vi "Graphical Test Runner - Main UI - .vi"() -> ()   [LabVIEW 2017]
doc: "Copyright © 2005 James Kring, Inc. - All Rights Reserved"
uses:
  Graphical Test Runner Support/Graphical TestRunner Throber List Static.ctl
  Graphical Test Runner Support/Graphical TestRunner Throber List Animated.ctl
  Classes/TestResult/resultStatusChanged--Cluster.ctl
  Classes/TestResult/resultStatus--enum.ctl
  Graphical Test Runner Support/FailbarStatus--Enum.ctl
  <userlib>/_OpenG.lib/comparison/comparison.llb/I32 Changed__ogtk.vi
  <userlib>/_OpenG.lib/file/file.llb/Valid Path - Traditional__ogtk.vi
  <userlib>/_OpenG.lib/array/array.llb/Filter 1D Array (Path)__ogtk.vi
  <userlib>/_OpenG.lib/file/file.llb/Strip Path - Arrays__ogtk.vi
  JKI Reuse/Filter Error Codes (Array)__jki_lib_error_handling -- VI Tester.vi
  <userlib>/_OpenG.lib/array/array.llb/Filter 1D Array (String)__ogtk.vi
  <userlib>/_OpenG.lib/array/array.llb/Delete Elements from 1D Array (Path)__ogtk.vi
  <userlib>/_OpenG.lib/array/array.llb/Conditional Auto-Indexing Tunnel (Path)__ogtk.vi
  <userlib>/_OpenG.lib/array/array.llb/Sort 1D Array (String)__ogtk.vi
  <userlib>/_OpenG.lib/array/array.llb/Index 1D Array Elements (Path)__ogtk.vi
  JKI Reuse/Filter Error Codes (Scalar)__jki_lib_error_handling -- VI Tester.vi
  Graphical Test Runner Support/GraphicalTestRunner.lvlib
  Libraries/VITesterUtilities.lvlib
  <vilib>/Utility/NIReport.llb/NI_report.lvclass
  Classes/TestResult/TestResult.lvclass
panel:
  in  "API_TesterStatus":refnum<user-event>
  in  "API_CompleteTestReport":refnum<user-event>
  in  "API_TextTestRunner":refnum<class>
  in  "Save Report":bool
  in  "API_TestObject":refnum<class>
  in  "Collapse Item":bool
  in  "Expand Item":bool
  in  "Collapse Tree":bool
  in  "Expand Tree":bool
  in  "Reload":bool
  in  "API_RunAll":bool
  in  "Abort":bool
  in  "Run Single Test":bool
  in  "Run All":bool
  out "Static Throber":T1=1
  out "Animated Throber":T2=1
  out "Slide":dbl(slide) min=0.0 max=100.0 scale=0.0..100.0
  out "txtRuns:":string caption="Last Run:"
  out "txtPassed:":string caption="Passed:"
  out "txtFailed:":string caption="Failed:"
  out "txtSkipped":string caption="Skipped:"
  in  "Test Hierarchy Tree":string(tree)
  out "Detailed Status":string
  out "Simple Status":string="Initializing ..."
  # "Copyright © 2007 James Kring, Inc. All rights reserved.\n\nAuthor: Omar Mussa [omar.mussa@jameskring.com]\n\nThis library is provided \"AS IS\" ,WITHOUT WARRANTIES OR \nCONDITIONS OF ANY KIND, either express or implied.\n\nJames Kring, Inc. -- http://www.jameskring.com"
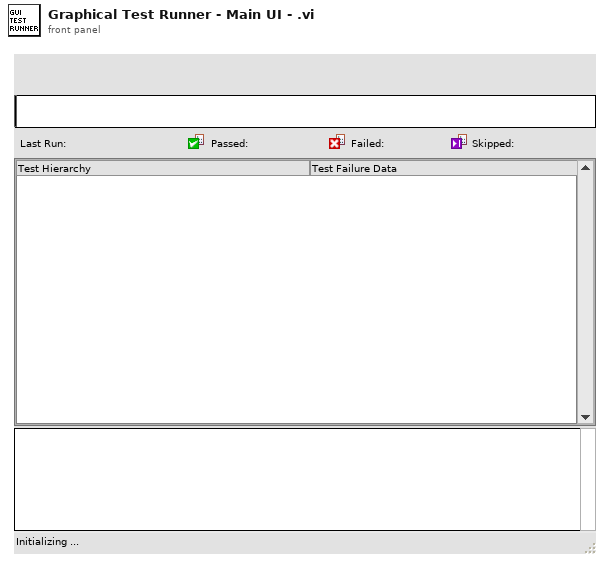
[diagram p1: front panel]
types:
  T1 = typedef "GraphicalTestRunner.lvlib/Graphical TestRunner Throber List Static.ctl" = u16
  T2 = typedef "GraphicalTestRunner.lvlib/Graphical TestRunner Throber List Animated.ctl" = u16
  T3 = typedef "TestResult.lvclass/resultStatusChanged--Cluster.ctl" = cluster{"test":refnum<class>, "resultStatus":T4, "TestResult":refnum<class>, "test error":errorcluster, "execution time (sec)":dbl}
  T4 = typedef "TestResult.lvclass/resultStatus--enum.ctl" = enum16{"testPass", "testFailure", "testError", "testSkipped"}
  T5 = cluster{"test":refnum<class>, "startTimestamp":timestamp}
  T6 = cluster{"Current VI's Refnum":refnum<vi>, "menubar":refnum<k9>, "TextStream":refnum<queue>, "StartTestTime":timestamp, "TestRunning":bool, "TestMethod":string, "Open Path":path, "Test Project":path, "TestProjectClasses":path[], "TestApplicationContext":refnum<vi>, "Test Class":path, "ResultChangedRef":refnum<user-event>, "SuiteChangedRef":refnum<user-event>, "TotalTests":i32, "TestTag":string, "Last Failure":string, "Last Tree Value":string, "AbortEventRef":refnum<user-event>, "TestMethods":path[], "ExitEventReference":refnum<user-event>, "InitializingTree":bool, "TestStartedEventRef":refnum<user-event>, "ProductName":string}
  T7 = cluster{"TestSuite":refnum<class>, "suiteStatus":enum16{"suiteStart", "suiteStop", "suiteSkip"}}
  T8 = enum8{"Enabled", "Disabled", "Disabled and Grayed Out"}
  T9 = enum32{"Invalid", "Standard", "Closed", "Hidden", "Minimized", "Maximized"}
  T10 = typedef "GraphicalTestRunner.lvlib/FailbarStatus--Enum.ctl" = enum16{"Initialize", "Start", "Update Progress", "Fail", "Pass"}
  T11 = cluster{"ResultStatusChanged":refnum<user-event>, "SuiteStatusChanged":refnum<user-event>, "Exit":refnum<user-event>, "Abort":refnum<user-event>, "TestStartedEventRef":refnum<user-event>}
  T12 = enum32{"existing file", "new file", "new or existing file", "existing dir", "new dir", "new or existing dir", "existing file (use LLBs)", "new file (use LLBs)", "new or existing file (use LLBs)", "new or existing file or directory (use LLBs)", "existing dir (use LLBs)", "new dir (use LLBs)", "new or existing dir (use LLBs)", "existing file or dir", "new file or dir", "new or existing file or dir", "existing file or dir (use LLBs)", "new file or dir (use LLBs)", "multi-select", "multi-select (use LLBs)"}
  T13 = typedef "LVPoint32TypeDef.ctl" = cluster{"Horizontal":i32, "Vertical":i32}
  T14 = cluster{"Recent Paths":path[], "SkipMassCompileCheck":bool}
  T15 = typedef "Filtered Error Details - Cluster__jki_lib_error_handling -- VI Tester.ctl" = cluster{"code":i32, "source":string}
  T16 = typedef "imagedata.ctl" = cluster{"image type":i32, "image depth":i32, "image":u8[], "mask":u8[], "colors":u32[], "Rectangle":cluster{"left":i16, "top":i16, "right":i16, "bottom":i16}}
  T17 = cluster{"txtRuns":refnum<vi>, "txtSkipped":refnum<vi>, "txtFailures":refnum<vi>, "txtPassed":refnum<vi>, "txtSimple Status":refnum<vi>, "Test Hierarchy Tree":refnum<vi>}
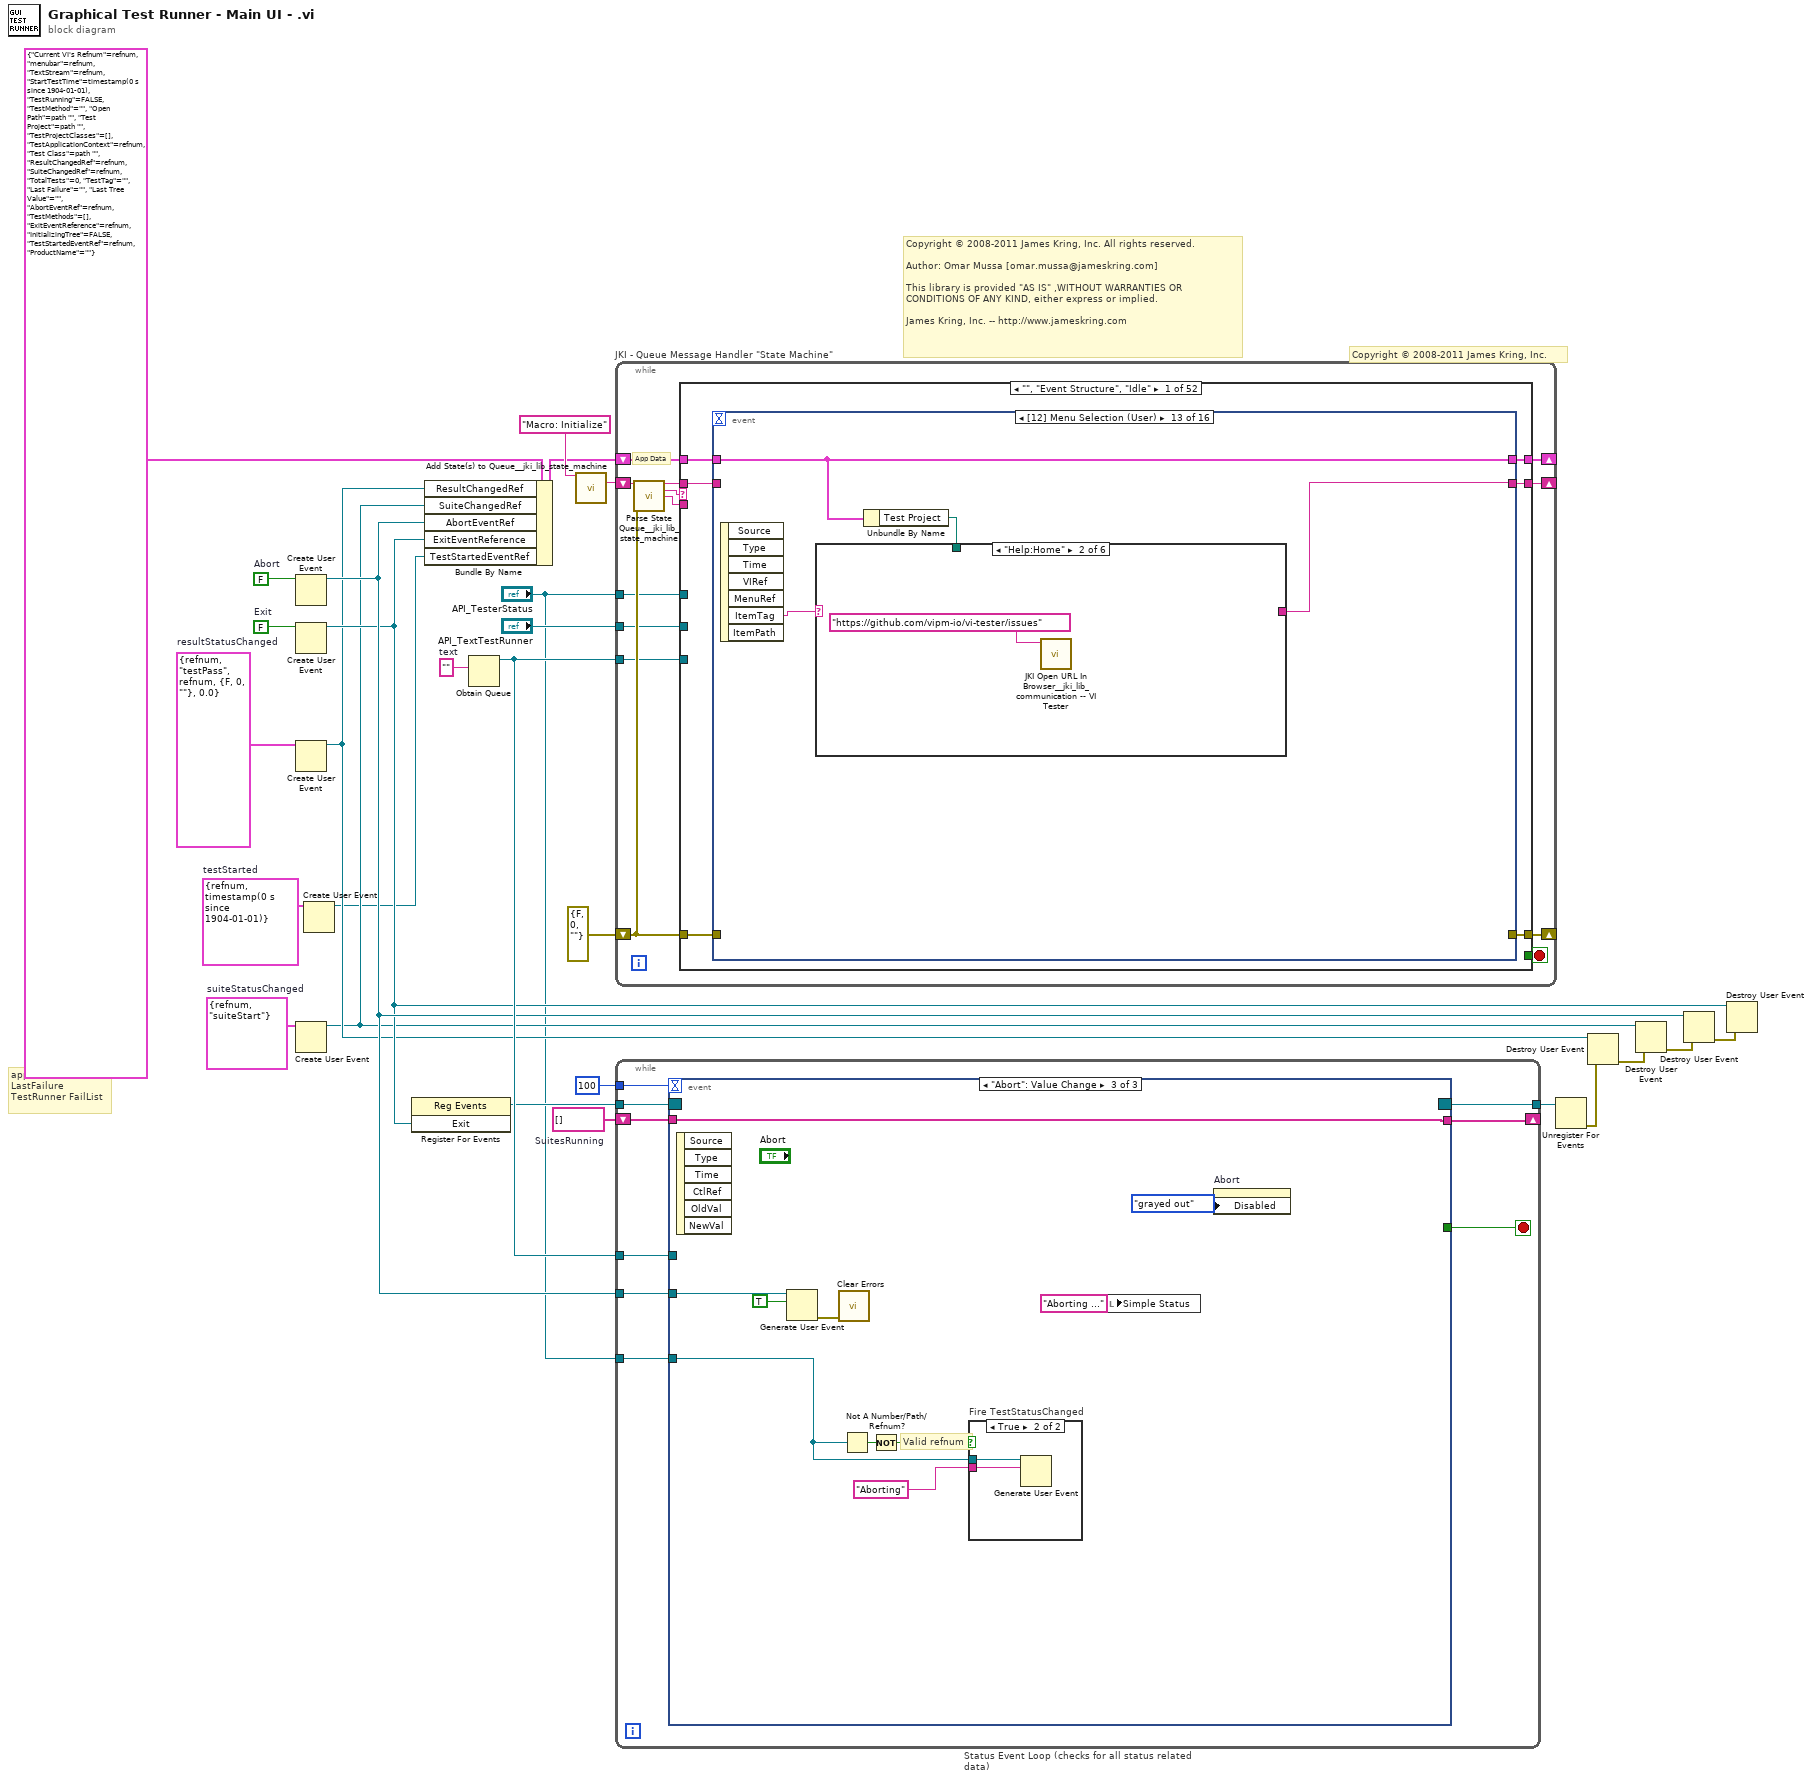
[diagram p0: block diagram]
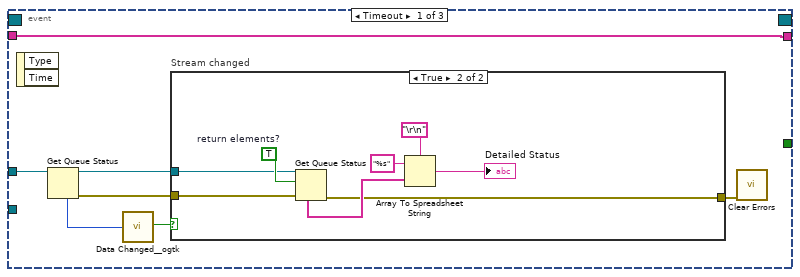
[diagram p2: hidden frame]
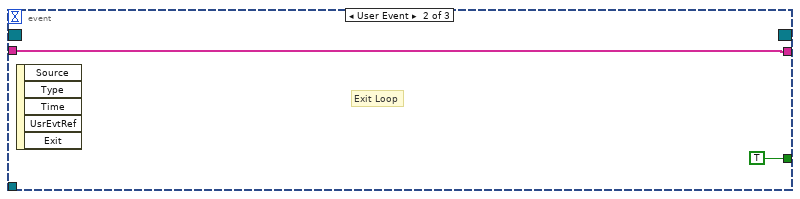
[diagram p4: hidden frame]
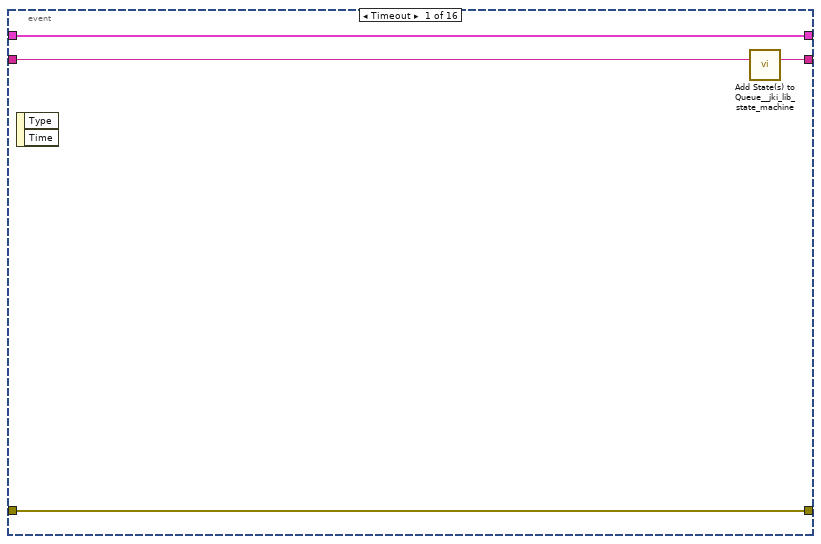
[diagram p6: hidden frame]
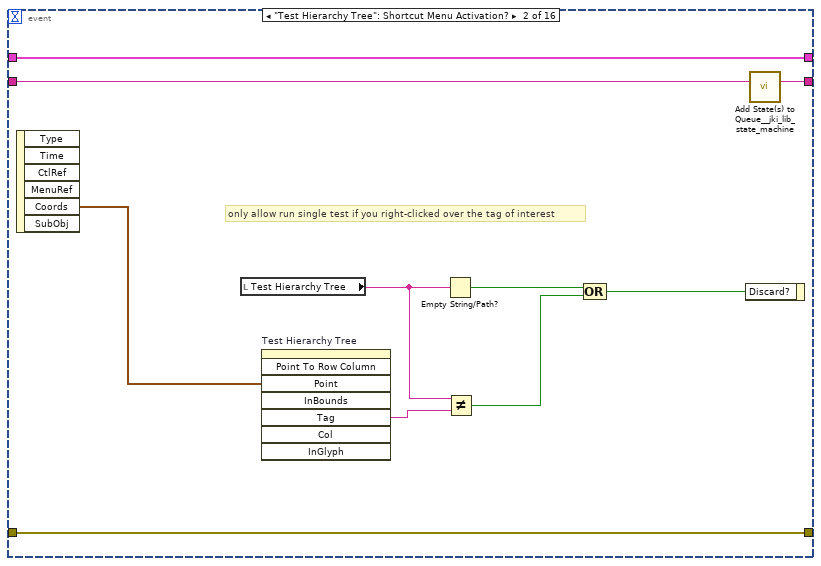
[diagram p7: hidden frame]
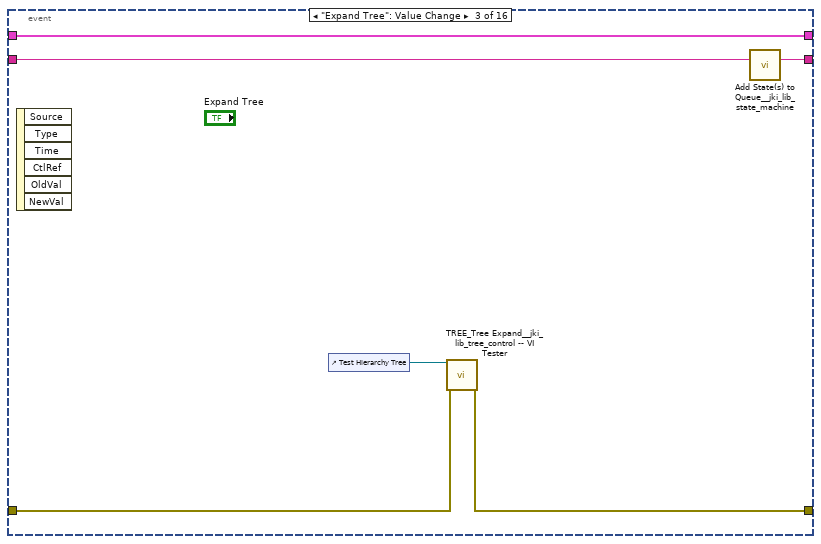
[diagram p8: hidden frame]
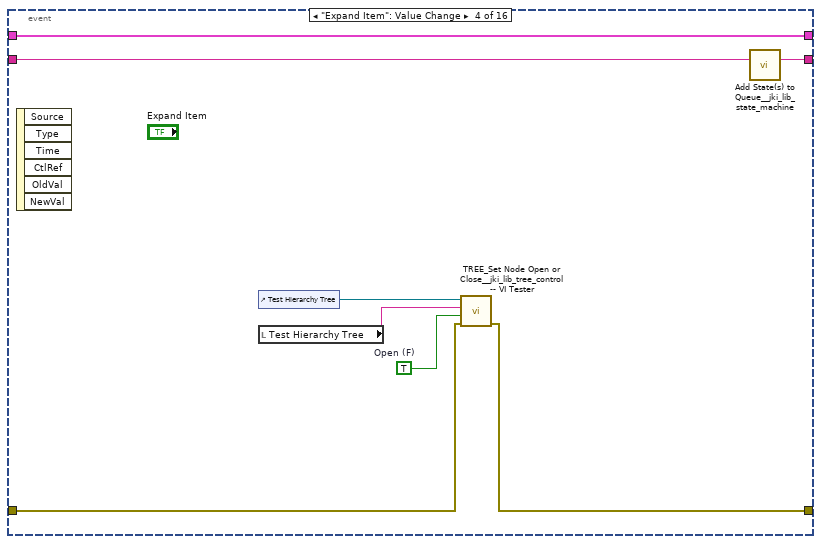
[diagram p9: hidden frame]
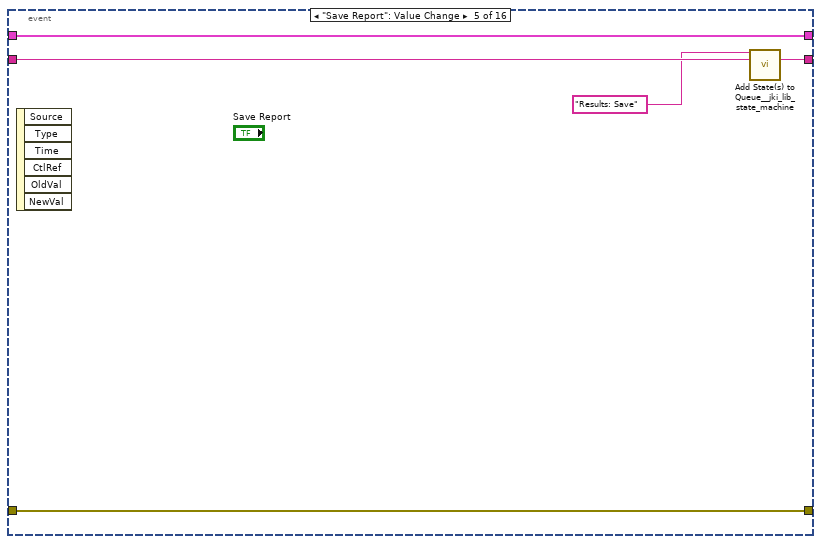
[diagram p10: hidden frame]
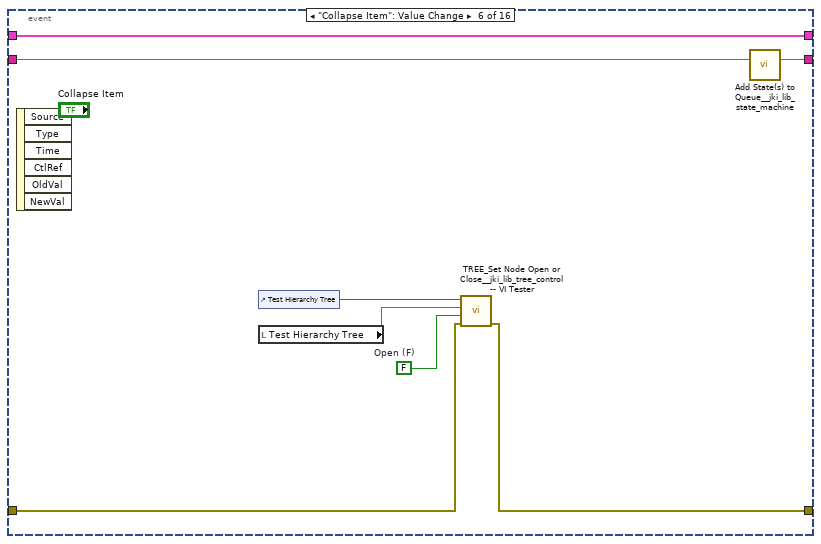
[diagram p11: hidden frame]
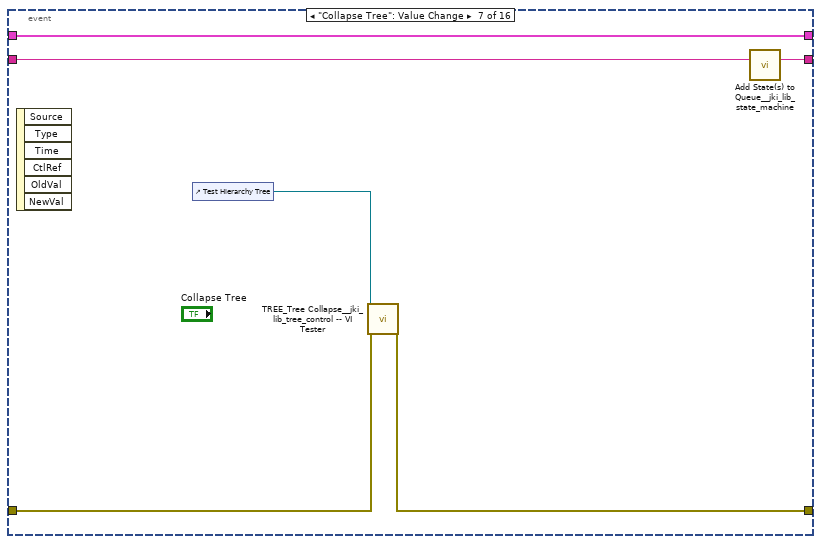
[diagram p12: hidden frame]
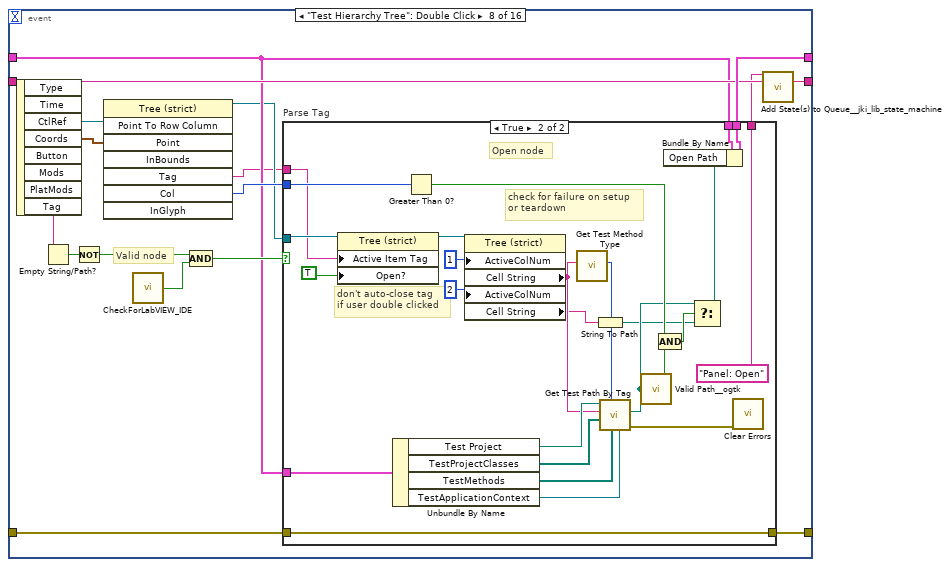
[diagram p13: hidden frame]
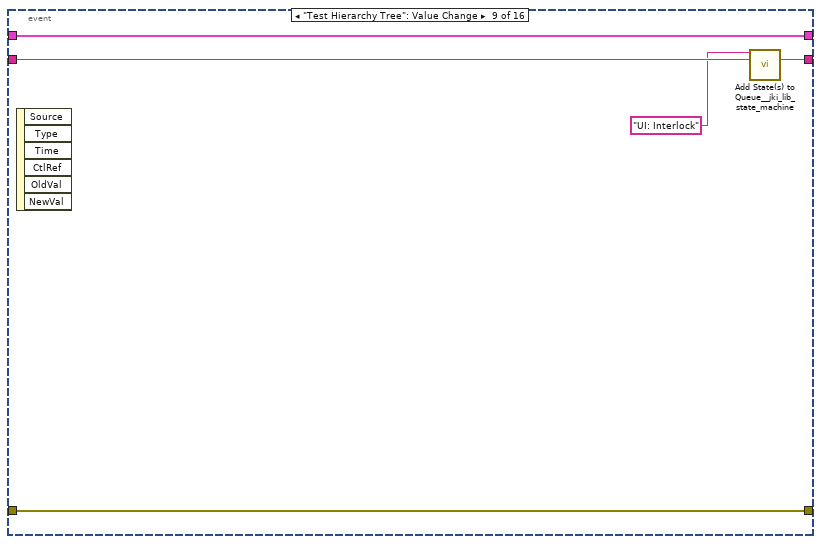
[diagram p15: hidden frame]
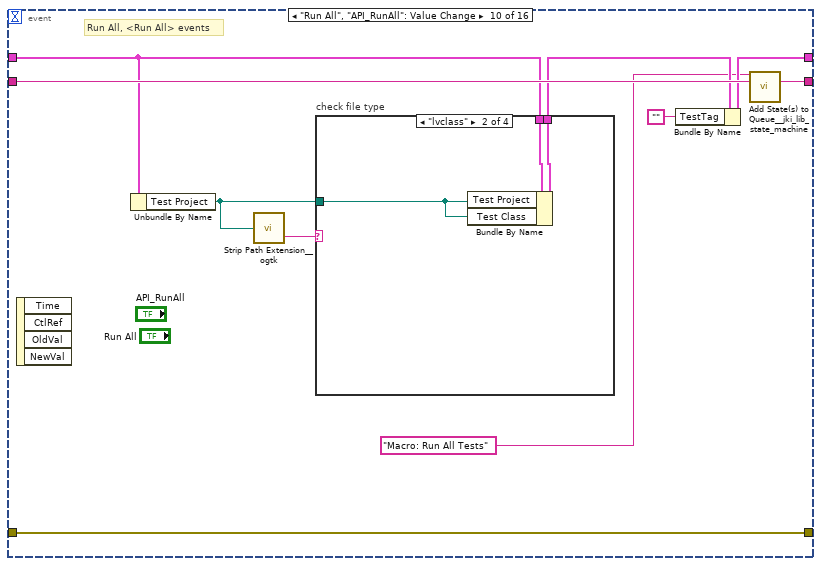
[diagram p16: hidden frame]
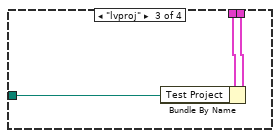
[diagram p18: hidden frame]
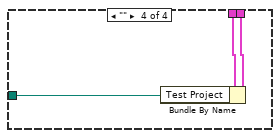
[diagram p19: hidden frame]
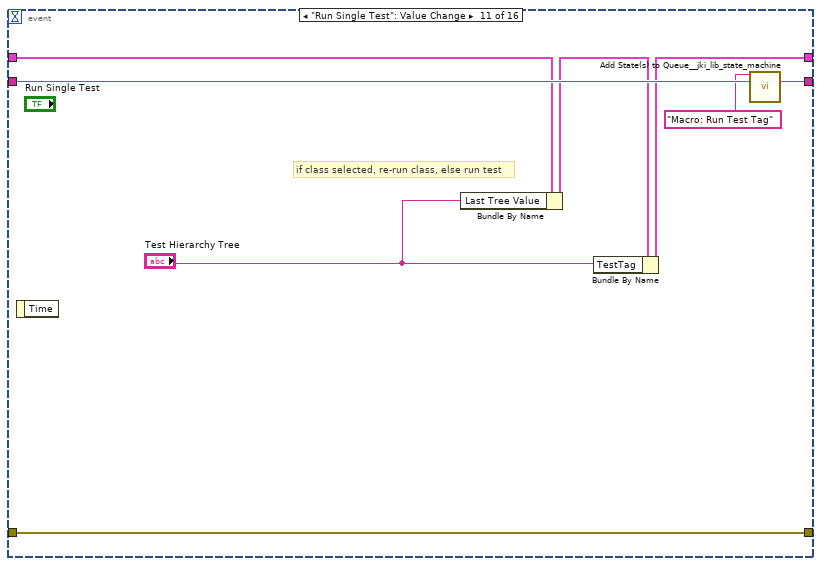
[diagram p20: hidden frame]
diagram:
  w2 = T3 {"test"=refnum, "resultStatus"=enum."testPass", "TestResult"=refnum, "test error"={"status"=FALSE, "code"=0, "source"=""}, "execution time (sec)"=0.0}  # resultStatusChanged
  w7 = T5 {"test"=refnum, "startTimestamp"=timestamp(0 s since 1904-01-01)}  # testStarted
  w8 = ""  # text
  w12 = FALSE  # Exit
  w16 = FALSE  # Abort
  w18 = string[] []  # SuitesRunning
  w19 = T7 {"TestSuite"=refnum, "suiteStatus"=enum."suiteStart"}  # suiteStatusChanged
  # "app data to delete\nLastFailure\nTestRunner FailList"
  # "Copyright © 2008-2011 James Kring, Inc. All rights reserved.\n\nAuthor: Omar Mussa [omar.mussa@jameskring.com]\n\nThis library is provided \"AS IS\" ,WITHOUT WARRANTIES OR \nCONDITIONS OF ANY KIND, either express or implied.\n\nJames Kring, Inc. -- http://www.jameskring.com"
  # "Copyright © 2008-2011 James Kring, Inc."
  n1 = Create User Event(user event datatype=w16) -> (user event=w13:refnum<user-event>)  [unwired: 1 in, 1 out]
  n2 = Create User Event(user event datatype=w12) -> (user event=w10:refnum<user-event>)  [unwired: 1 in, 1 out]
  n3 = Create User Event(user event datatype=w2) -> (user event=w6:refnum<user-event>)  [unwired: 1 in, 1 out]
  n4 = Create User Event(user event datatype=w19) -> (user event=w5:refnum<user-event>)  [unwired: 1 in, 1 out]
  n5 = Create User Event(user event datatype=w7) -> (user event=w4:refnum<user-event>)  [unwired: 1 in, 1 out]
  n6 = register-events(w10) -> (reference out=w22:refnum<event-registration>)  [unwired: 2 in, 1 out]
  n7 = Bundle By Name(cluster=T6 {"Current VI's Refnum"=refnum, "menubar"=refnum, "TextStream"=refnum, "StartTestTime"=timestamp(0 s since 1904-01-01), "TestRunning"=FALSE, "TestMethod"="", "Open Path"=path "", "Test Project"=path "", "TestProjectClasses"=[], "TestApplicationContext"=refnum, "Test Class"=path "", "ResultChangedRef"=refnum, "SuiteChangedRef"=refnum, "TotalTests"=0, "TestTag"="", "Last Failure"="", "Last Tree Value"="", "AbortEventRef"=refnum, "TestMethods"=[], "ExitEventReference"=refnum, "InitializingTree"=FALSE, "TestStartedEventRef"=refnum, "ProductName"=""} ("SMUI Template App Data"), "ResultChangedRef"=w6, "SuiteChangedRef"=w5, "AbortEventRef"=w13, "ExitEventReference"=w10, "TestStartedEventRef"=w4) -> (w23:T6)
  n8 = Obtain Queue(element data type=w8) -> (queue out=w24:refnum<queue>)  [unwired: 4 in, 2 out]
  n9 = call <vilib>:"Add State(s) to Queue__jki_lib_state_machine.vi"("State(s) in Front (\"\")"="Macro: Initialize") -> ("States Out"=w26:string)  [unwired: 14 in]
  n10 = while "JKI - Queue Message Handler \"State Machine\"" {
    shift-right: [w40] -> _
    shift-left: errorcluster {"status"=FALSE, "code"=0, "source"=""} ("error out") -> [w34]
    shift-right: [w38] -> _
    shift-left: w26 -> [w35]
    shift-right: [w36] -> _
    shift-left: w23 -> [w37]
    tunnel: w24 -> [w30]
    tunnel: "API_TextTestRunner" -> [w29]
    tunnel: "API_TesterStatus" -> [w28]
    stop <- w39 stop-if-true
    # "App Data"
    n11 = call <vilib>:"Parse State Queue__jki_lib_state_machine.vi"("State Queue"=w35, "Error In (no error)"=w34) -> ("Remaining States"=w33:string, "Current State"=w31:string, "Arguments"=w32:string)  [unwired: 11 in]
    n12 = case shown="\"\", \"Event Structure\", \"Idle\"" w31 {
      selector: w31 -> [_ _ w261 _ _ _ _ _ _ _ _ _ _ _ _ _ _ _ _ _ _ _ _ _ _ _ _ _ _ _ _ _ _ _ _ _ _ _ _ _ _ _ _ _ _ _ _ _ _ _ _ _]
      tunnel: w33 -> [w45 w252 w259 w270 w291 w305 w325 w333 w354 w357 w367 w376 w387 w405 w441 w447 w465 w477 w492 w523 w526 w537 w587 w609 w613 w628 w644 w659 w670 w680 w704 w723 w726 w734 w745 w756 w771 w804 w811 w828 w837 w842 w847 w857 w861 w872 w876 w889 w901 w910 w929 w939]
      tunnel: [w42 w254 w255 errorcluster {"status"=FALSE, "code"=0, "source"=""} ("error out") w293 w300 w327 w328 w334 w359 w361 w369 w378 w402 w442 w448 w467 w479 w494 w514 w528 w530 w589 w598 w610 w621 w629 w660 w667 w678 w688 w724 w728 w729 w735 w758 w767 w792 w813 w814 w839 w844 w849 w858 w863 w874 w878 w890 w903 w905 w918 w941] -> w40
      tunnel: w34 -> [w41 w254 _ w268 w293 w297 w327 w329 w334 w359 w361 w369 w383 w402 w442 w448 w467 w479 w494 w515 w528 w531 w589 w599 w610 w616 w630 w660 w666 w675 w682 w724 w728 w730 w735 w758 w769 w793 w813 w814 w839 w844 w849 w858 w863 w874 w878 w890 w903 w907 w919 w941]
      tunnel: [_ _ _ _ TRUE _ _ _ _ _ _ _ _ _ _ _ _ _ _ _ _ _ _ _ _ _ _ _ _ _ _ _ _ _ _ _ _ _ _ _ _ _ _ _ _ _ _ _ _ _ _ _] -> w39
      tunnel: [w46 w251 w260 w269 w291 w305 w324 w332 w353 w356 w366 w375 w386 w404 w440 w446 w466 w478 w493 w524 w525 w536 w586 w608 w612 w627 w643 w658 w669 w679 w703 w722 w725 w733 w744 w756 w770 w803 w810 w827 w836 w841 w846 w856 w860 w871 w875 w888 w900 w909 w928 w938] -> w38
      tunnel: w37 -> [w44 w253 w258 w263 w290 w299 w326 w331 w343 w358 w368 w377 w385 w406 w438 w445 w464 w476 w482 w522 w527 w533 w588 w600 w611 w614 w645 w655 w668 w673 w702 w715 w727 w732 w740 w757 w766 w801 w812 w826 w838 w843 w848 w855 w862 w873 w877 w884 w902 w911 w915 w940]
      tunnel: [w43 w253 w258 w263 w290 w299 w326 w331 w355 w358 w368 w377 w385 w406 w438 w445 w464 w476 w481 w522 w527 w533 w588 w600 w611 w626 w642 w655 w668 w673 w702 w721 w727 w732 w737 w757 w768 w802 w812 w818 w838 w843 w848 w855 w862 w873 w877 w883 w902 w911 w915 w940] -> w36
      tunnel: w32 -> [_ _ _ _ _ _ _ _ _ _ _ _ _ _ _ w444 _ _ _ _ _ _ _ _ _ _ _ w657 _ _ _ _ _ _ w743 _ _ _ _ _ _ _ _ _ _ _ _ _ _ _ _ _]
      tunnel: w30 -> [_ _ _ _ _ _ _ _ w344 _ _ _ _ _ _ _ w453 _ _ _ _ _ _ _ _ _ w635 _ _ _ w692 _ _ _ _ _ _ _ _ _ _ _ _ _ _ _ _ _ _ _ _ _]
      tunnel: w29 -> [_ _ _ _ _ _ _ _ _ _ _ _ _ _ _ _ _ _ _ _ _ _ _ _ _ w615 _ _ w665 w672 _ _ _ _ _ _ _ _ _ _ _ _ _ _ _ _ _ _ _ _ _ _]
      tunnel: w28 -> [_ _ _ _ _ _ _ _ _ _ _ _ _ _ _ _ _ _ _ _ _ _ _ _ _ _ w631 _ _ _ w684 _ _ _ _ _ _ _ _ _ _ _ _ _ _ _ _ _ _ _ _ _]
      frame "", "Event Structure", "Idle" {
        n13 = event shown="[12] Menu Selection (User)" {
          selector: _ -> [_ _ _ _ _ _ _ _ _ _ _ _ _ _ _ _]
          dyn-events: _ -> [_ _ _ _ _ _ _ _ _ _ _ _ _ _ _ _]
          timeout: _ -> [_ _ _ _ _ _ _ _ _ _ _ _ _ _ _ _]
          tunnel: [w49 w59 w65 w73 w78 w86 w92 w106 w142 w152 w170 w177 w186 _ w235 "Macro: Exit"] -> w46
          tunnel: w45 -> [w50 w60 w66 w74 w79 w87 w93 w107 w143 w153 w171 w178 _ _ _ _]
          tunnel: w44 -> [w48 w58 w64 w72 w77 w85 w91 w97 w141 w147 w165 w175 w184 w224 w233 w249]
          tunnel: [w48 w58 w64 w72 w77 w85 w91 w110 w141 w149 w169 w173 w184 w224 w232 w249] -> w43
          tunnel: [w47 w57 w61 w69 w76 w82 w88 w109 w140 w144 w167 w176 _ w220 _ _] -> w42
          tunnel: w41 -> [w47 w57 w62 w70 w76 w83 w89 w96 w140 w144 w167 w176 _ w222 _ _]
          event Timeout {
            n14 = event-data() -> ()  [unwired: 1 in, 2 out]
            n15 = call <vilib>:"Add State(s) to Queue__jki_lib_state_machine.vi"("State(s) in (\"\")"=w50) -> ("States Out"=w49:string)  [unwired: 14 in]
          }
          event "Test Hierarchy Tree": Shortcut Menu Activation? {
            # "only allow run single test if you right-clicked over the tag of interest"
            n16 = event-data() -> ("Coords"=w53:T13)  [unwired: 1 in, 5 out]
            n17 = local read "Test Hierarchy Tree"() -> (w51:string)
            n18 = invoke on="Test Hierarchy Tree" class="Tree (strict)" method="Point To Row Column"("Point"=w53) -> ("Tag"=w52:string)  [unwired: 7 in, 7 out]
            n19 = Empty String/Path?(string/path=w51) -> (empty?=w55:bool)
            n20 = Not Equal?(x=w51, y=w52) -> (x != y?=w56:bool)
            n21 = Compound Arithmetic op=OR(w55, w56) -> (w54:bool)
            n22 = event-data("Discard?"=w54) -> ()  [unwired: 1 in, 1 out]
            n23 = call <vilib>:"Add State(s) to Queue__jki_lib_state_machine.vi"("State(s) in (\"\")"=w60) -> ("States Out"=w59:string)  [unwired: 14 in]
          }
          event "Expand Tree": Value Change {
            n24 = event-data() -> ()  [unwired: 1 in, 6 out]
            n25 = control-ref of="Test Hierarchy Tree"() -> (w63:refnum<vi>)
            n26 = call "TREE_Tree Expand__jki_lib_tree_control -- VI Tester.vi"("Tree Reference In"=w63, "error in (no error)"=w62) -> ("error out"=w61:errorcluster)  [unwired: 16 in, 1 out]
            n27 = call <vilib>:"Add State(s) to Queue__jki_lib_state_machine.vi"("State(s) in (\"\")"=w66) -> ("States Out"=w65:string)  [unwired: 14 in]
          }
          event "Expand Item": Value Change {
            w67 = TRUE  # Open (F)
            n28 = event-data() -> ()  [unwired: 1 in, 6 out]
            n29 = control-ref of="Test Hierarchy Tree"() -> (w71:refnum<vi>)
            n30 = local read "Test Hierarchy Tree"() -> (w68:string)
            n31 = call "TREE_Set Node Open or Close__jki_lib_tree_control -- VI Tester.vi"("error in (no error)"=w70, "Open (F)"=w67, "Tag"=w68, "Tree Reference In"=w71) -> ("error out"=w69:errorcluster)  [unwired: 5 in, 2 out]
            n32 = call <vilib>:"Add State(s) to Queue__jki_lib_state_machine.vi"("State(s) in (\"\")"=w74) -> ("States Out"=w73:string)  [unwired: 14 in]
          }
          event "Save Report": Value Change {
            n33 = event-data() -> ()  [unwired: 1 in, 6 out]
            n34 = call <vilib>:"Add State(s) to Queue__jki_lib_state_machine.vi"("State(s) in Front (\"\")"="Results: Save" ("State(s) in Front (\"\")"), "State(s) in (\"\")"=w79) -> ("States Out"=w78:string)  [unwired: 13 in]
          }
          event "Collapse Item": Value Change {
            w80 = FALSE  # Open (F)
            n35 = event-data() -> ()  [unwired: 1 in, 6 out]
            n36 = control-ref of="Test Hierarchy Tree"() -> (w84:refnum<vi>)
            n37 = local read "Test Hierarchy Tree"() -> (w81:string)
            n38 = call "TREE_Set Node Open or Close__jki_lib_tree_control -- VI Tester.vi"("error in (no error)"=w83, "Open (F)"=w80, "Tag"=w81, "Tree Reference In"=w84) -> ("error out"=w82:errorcluster)  [unwired: 5 in, 2 out]
            n39 = call <vilib>:"Add State(s) to Queue__jki_lib_state_machine.vi"("State(s) in (\"\")"=w87) -> ("States Out"=w86:string)  [unwired: 14 in]
          }
          event "Collapse Tree": Value Change {
            n40 = event-data() -> ()  [unwired: 1 in, 6 out]
            n41 = control-ref of="Test Hierarchy Tree"() -> (w90:refnum<vi>)
            n42 = call "TREE_Tree Collapse__jki_lib_tree_control -- VI Tester.vi"("Tree Reference In"=w90, "error in (no error)"=w89) -> ("error out"=w88:errorcluster)  [unwired: 16 in, 1 out]
            n43 = call <vilib>:"Add State(s) to Queue__jki_lib_state_machine.vi"("State(s) in (\"\")"=w93) -> ("States Out"=w92:string)  [unwired: 14 in]
          }
          event "Test Hierarchy Tree": Double Click {
            # "Valid node"
            n44 = event-data() -> ("CtlRef"=w100:refnum<vi>, "Coords"=w99:T13, "Tag"=w101:string)  [unwired: 1 in, 5 out]
            n45 = Empty String/Path?(string/path=w101) -> (empty?=w108:bool)
            n46 = Not(x=w108) -> (.not. x?=w104:bool)
            n47 = invoke class="Tree (strict)" method="Point To Row Column"(reference=w100, "Point"=w99) -> (reference out=w95:refnum<vi>, "Tag"=w94:string, "Col"=w98:i32)  [unwired: 6 in, 5 out]
            n48 = call "CheckForLabVIEW_IDE.vi"() -> ("LabVIEW IDE"=w102:bool)
            n49 = Compound Arithmetic op=AND(w104, w102) -> (w103:bool)
            n50 = case "Parse Tag" shown="True" w103 {
              tunnel: [w111 w138] -> w110
              tunnel: [w112 w113] -> w109
              tunnel: w97 -> [w111 w137]
              tunnel: w96 -> [w112 w113]
              tunnel: [_ "Panel: Open" ("State(s) in Front")] -> w105
              tunnel: w98 -> [_ w135]
              tunnel: w95 -> [_ w120]
              tunnel: w97 -> [_ w133]
              tunnel: w94 -> [_ w117]
              frame False {
                # "Ignore double click if:\n1) Invalid node selected\n2) Running from Built EXE"
              }
              frame True {
                # "don't auto-close tag\nif user double clicked"
                # "check for failure on setup\nor teardown"
                # "Open node"
                n51 = property class="Tree (strict)"(reference=w120, "Active Item Tag"=w117, "Open?"=TRUE ("Active Item:Open?")) -> (reference out=w119:refnum<vi>)  [unwired: 1 in, 1 out]
                n52 = Unbundle By Name(w133) -> ("Test Project"=w132:path, "TestProjectClasses"=w129:path[], "TestMethods"=w128:path[], "TestApplicationContext"=w127:refnum<vi>)
                n53 = Greater Than 0?(x=w135) -> (x > 0?=w126:bool)
                n54 = property class="Tree (strict)"(reference=w119, "ActiveColNum"=1 ("Active Cell:Active Column Number"), "ActiveColNum"=2 ("Active Cell:Active Column Number")) -> ("Cell String"=w131:string, "Cell String"=w115:string)  [unwired: 1 in, 2 out]
                n55 = call "Get Test Method Type.vi"("Failure String"=w131) -> ("method type"=w130:enum16{"setUp", "testMethod", "tearDown"})  [unwired: 10 in]
                n56 = String To Path(string=w115) -> (path=w114:path)
                n57 = call "Get Test Path By Tag.vi"("TestApplicationContext"=w127, "TestMethods"=w128, "Method (testMethod)"=w130, "TestProjectClasses"=w129, "TestMethod Tag"=w131, "Test Project"=w132) -> ("error out"=w121:errorcluster, "Path"=w123:path)  [unwired: 2 in, 2 out]
                n58 = call-poly <userlib>:"Valid Path__ogtk.vi"("path"=w123) -> ("valid"=w125:bool)
                n59 = Compound Arithmetic op=AND(w126, w125) -> (w124:bool)
                n60 = Select(t=w123, s=w124, f=w114) -> (s? t:f=w122:path)
                n61 = Bundle By Name(cluster=w137, "Open Path"=w122) -> (w138:T6)
                n62 = call <vilib>:"Clear Errors.vi"("error in (no error)"=w121) -> ()  [unwired: 5 in, 2 out]
              }
            }
            n63 = call <vilib>:"Add State(s) to Queue__jki_lib_state_machine.vi"("State(s) in Front (\"\")"=w105, "State(s) in (\"\")"=w107) -> ("States Out"=w106:string)  [unwired: 13 in]
          }
          event "Test Hierarchy Tree": Value Change {
            n64 = event-data() -> ()  [unwired: 1 in, 6 out]
            n65 = call <vilib>:"Add State(s) to Queue__jki_lib_state_machine.vi"("State(s) in Front (\"\")"="UI: Interlock" ("State(s) in Front"), "State(s) in (\"\")"=w143) -> ("States Out"=w142:string)  [unwired: 13 in]
          }
          event "Run All", "API_RunAll": Value Change {
            # "Run All, <Run All> events"
            n66 = event-data() -> ()  [unwired: 1 in, 4 out]
            n67 = Unbundle By Name(w147) -> ("Test Project"=w145:path)
            n68 = call-poly <userlib>:"Strip Path Extension__ogtk.vi"("path"=w145) -> ("extension"=w150:string)  [unwired: 1 out]
            n69 = case "check file type" shown="\"lvclass\"" w150 {
              tunnel: w147 -> [w154 w157 w160 w163]
              tunnel: [w154 w156 w159 w162] -> w151
              tunnel: w145 -> [_ w155 w158 w161]
              frame Default {
              }
              frame "lvclass" {
                n70 = Bundle By Name(cluster=w157, "Test Project"=w155, "Test Class"=w155) -> (w156:T6)
              }
              frame "lvproj" {
                n71 = Bundle By Name(cluster=w160, "Test Project"=w158) -> (w159:T6)
              }
              frame "" {
                n72 = Bundle By Name(cluster=w163, "Test Project"=w161) -> (w162:T6)
              }
            }
            n73 = Bundle By Name(cluster=w151, "TestTag"="") -> (w149:T6)
            n74 = call <vilib>:"Add State(s) to Queue__jki_lib_state_machine.vi"("State(s) in Front (\"\")"="Macro: Run All Tests", "State(s) in (\"\")"=w153) -> ("States Out"=w152:string)  [unwired: 13 in]
          }
          event "Run Single Test": Value Change {
            # "if class selected, re-run class, else run test"
            n75 = event-data() -> ()  [unwired: 1 in, 1 out]
            n76 = Bundle By Name(cluster=w165, "Last Tree Value"="Test Hierarchy Tree") -> (w164:T6)
            n77 = Bundle By Name(cluster=w164, "TestTag"="Test Hierarchy Tree") -> (w169:T6)
            n78 = call <vilib>:"Add State(s) to Queue__jki_lib_state_machine.vi"("State(s) in Front (\"\")"="Macro: Run Test Tag", "State(s) in (\"\")"=w171) -> ("States Out"=w170:string)  [unwired: 13 in]
          }
          event "Test Hierarchy Tree": Shortcut Menu Selection (User) {
            n79 = event-data() -> ("ItemTag"=w174:string)  [unwired: 1 in, 5 out]
            n80 = case "Get Selected Method" shown="\"RunSingleTest\"" w174 {
              tunnel: w175 -> [w182 w183]
              tunnel: [w181 w183] -> w173
              tunnel: ["Macro: Run Test Tag" _] -> w172
              frame "RunSingleTest" {
                # "if class selected, re-run class, else run test"
                n81 = local read "Test Hierarchy Tree"() -> (w179:string)
                n82 = Bundle By Name(cluster=w182, "Last Tree Value"=w179, "TestTag"=w179) -> (w181:T6)
              }
              frame Default {
              }
            }
            n83 = call <vilib>:"Add State(s) to Queue__jki_lib_state_machine.vi"("State(s) in Front (\"\")"=w172, "State(s) in (\"\")"=w178) -> ("States Out"=w177:string)  [unwired: 13 in]
          }
          event Menu Selection (User) {
            n84 = event-data() -> ("ItemTag"=w187:string)  [unwired: 1 in, 6 out]
            n85 = Unbundle By Name(w184) -> ("Test Project"=w185:path)
            n86 = case shown="\"Help:Home\"" w187 {
              selector: w187 -> [w189 _ _ _ _ _]
              tunnel: [w190 _ _ "Macro: Exit" _ "UI: Open File Dialog"] -> w186
              tunnel: w185 -> [_ _ _ _ w201 _]
              frame Default {
                n87 = call <userlib>:"Search or Split String__ogtk.vi"("search string/char (-)"="Recent_Files:", "string"=w189) -> ("offset after match"=w192:i32, "substring after match"=w188:string)  [unwired: 1 in, 1 out]
                n88 = Greater Or Equal To 0?(x=w192) -> (x >= 0?=w191:bool)
                n89 = case shown="True" w191 {
                  tunnel: [w194 w195] -> w190
                  tunnel: w189 -> [w194 _]
                  tunnel: w188 -> [_ w197]
                  frame False {
                  }
                  frame True {
                    n90 = Format Into String(format string="Project: Open >> %s", w197) -> (resulting string=w195:string)  [unwired: 2 in, 1 out]
                  }
                }
              }
              frame "Help:Home" {
                n91 = call "JKI Open URL In Browser__jki_lib_communication -- VI Tester.vi"("url"="https://github.com/vipm-io/vi-tester/issues") -> ()  [unwired: 5 in, 2 out]
              }
              frame "About VI Tester..." {
                n92 = call "VI Tester About.vi"() -> ()  [unwired: 1 in]
              }
              frame "Exit" {
              }
              frame "Estimate Coverage..." {
                # "Estimate Test Coverage - Main UI - .vi"
                n93 = Build Path(base path=w201, name or relative path="..\\Tests") -> ()  [unwired: 1 out]
              }
              frame "File:Open_Project" {
              }
            }
          }
          event Menu Activation? {
            w217 = "Recent_Files" ("menu tag")
            # "Keep only if exists on disk"
            # "rebuild menu"
            # "flush existing menu"
            n94 = event-data() -> ("MenuRef"=w215:refnum<k9>)  [unwired: 1 in, 5 out]
            n95 = call "Read General Settings.vi"("error in"=w222) -> ("error out"=w211:errorcluster, "General"=w221:T14)  [unwired: 9 in]
            n96 = Unbundle By Name(w221) -> ("Recent Paths"=w205:path[])
            n97 = Build Array(path "", path "") -> (w208:path[])
            n98 = call-poly <userlib>:"Filter 1D Array__ogtk.vi"("items to filter"=w208, "array"=w205) -> ("filtered array"=w204:path[])  [unwired: 4 in, 1 out]
            n99 = for {
              tunnel: w204 -> [w228] mode=indexing
              tunnel: [w227] -> w203 mode=indexing if=w225
              n100 = call <vilib>:"Librarian Get Info.vi"("path"=w228) -> ("error out"=w226:errorcluster, "dup path"=w227:path)  [unwired: 8 in, 1 out]
              n101 = Not(x=w226) -> (.not. x?=w225:bool)
            }
            n102 = call-poly <userlib>:"Strip Path__ogtk.vi"("path"=w203) -> ("name"=w219:string[])  [unwired: 1 out]
            n103 = for {
              tunnel: w203 -> [w231] mode=indexing
              tunnel: [w230] -> w209 mode=indexing
              tunnel: "Recent_Files:%s" ("menu tag") -> [w229]
              n104 = Format Into String(format string=w229, w231) -> (resulting string=w230:string)  [unwired: 2 in, 1 out]
            }
            n105 = Get Menu Item Info(7:w217, 8:w211, 11:w215) -> (0:w212:errorcluster, 3:w214:refnum<k9>, 5:w216:string[])  [unwired: 4 out]
            n106 = Delete Menu Items(6:w212, 7:w216, 8:w217, 9:w214) -> (0:w210:errorcluster, 3:w213:refnum<k9>)
            n107 = Insert Menu Items(5:w217, 6:w210, 7:w209, 8:w219, 9:w213) -> (0:w220:errorcluster)  [unwired: 1 in, 2 out]
            n108 = event-data("Discard?"=FALSE) -> ()  [unwired: 1 in, 1 out]
          }
          event "Reload": Value Change {
            # "Reload"
            n109 = event-data() -> ()  [unwired: 1 in, 6 out]
            n110 = Unbundle By Name(w233) -> ("StartTestTime"=w236:timestamp)
            n111 = Not Equal?(x=timestamp(0 s since 1904-01-01) ("y"), y=w236) -> (x != y?=w238:bool)
            n112 = case "Test results exist" shown="True" w238 {
              tunnel: [TRUE ("T button?") w246] -> w234
              frame False {
              }
              frame True {
                n113 = Two Button Dialog(message="Reloading will clear the current results.", 2:"Reload" ("T button name (\"OK\")")) -> (T button?=w246:bool)  [unwired: 1 in]
              }
            }
            n114 = case shown="True" w234 {
              tunnel: [_ "UI: Set Busy\nMacro: Load Tree\nUI: Set Free" ("message")] -> w235
              tunnel: w233 -> [w239 w242]
              tunnel: [w239 w241] -> w232
              frame False {
              }
              frame True {
                n115 = Bundle By Name(cluster=w242, "StartTestTime"=timestamp(0 s since 1904-01-01)) -> (w241:T6)
              }
            }
          }
          event Panel Close? {
            n116 = event-data() -> ()  [unwired: 1 in, 4 out]
            n117 = event-data("Discard?"=TRUE) -> ()  [unwired: 1 in, 1 out]
          }
        }
      }
      frame "---------- Core ----------" {
        n118 = call <vilib>:"Add State(s) to Queue__jki_lib_state_machine.vi"("State(s) in (\"\")"=w252) -> ("States Out"=w251:string)  [unwired: 14 in]
      }
      frame Default {
        w257 = 42 items=["No error", "Argument error", "Memory is full", "Out of zone", "End of file", "File already open", "Generic file I/O error", "File not found", "File permission error", "Disk is full", "Duplicate path", "Too many files open", "System feature not enabled", "Resource file not found", "Cannot add resource", "Resource not found", "Image not found", "Image memory error", "Pen does not exist", "Config type invalid", "Config token not found", "Config parse error", "Config memory error", "Bad external code format", "Bad external code offset", "External code not present", "Null window", "Destroy window error", "Null menu", "Print aborted", "Bad print record", "Print driver error", "Windows error during printing", "Memory error during printing", "Print dialog error", "Generic print error", "Invalid device refnum", "Device not found", "Device parameter error", "Device unit error", "Cannot open device", "Device call aborted", "Generic error", "Cancelled by user", "Object ID too low", "Object ID too high", "Object not in heap", "Unknown heap", "Unknown object (invalid DefProc)", "Unknown object (DefProc not in table)", "Message out of range", "Invalid (null) method", "Unknown message", "Manager call not supported", "Bad address", "Network operation in progress", "Network operation timed out", "Connection is busy", "Network attribute not supported", "Network error", "Address in use", "System out of memory", "Connection aborted", "Connection refused", "Not connected", "Already connected", "Connection closed", "Initialization error (interapplication manager)", "Bad occurrence", "Wait on unbound occurrence handler", "Occurrence queue overflow", "Datalog type conflict", "Unused", "Unrecognized type (interapplication manager)", "Memory corrupt", "Failed to make temporary DLL", "Old CIN version", "Drag socket not found", "Failed to load drop-object", "Failed to register OLE object", "Failed to release OLE object", "Format specifier type mismatch", "Unknown format specifier", "Too few format specifiers", "Too many format specifiers", "Scan failed", "Newer CIN version", "Error converting to variant", "Runtime menu error", "Password tampered", "Variant attribute not found", "Incompatible variant data type", "Event data is not available", "Event Store is not present", "Occurrence is not found", "Event Queue is not created", "Event info is not available", "Refnum passed is NULL", "Error retrieving Class GUID", "Error retrieving CoClass GUID", "Error retrieving TypeLib GUID.", "Bad built application magic bytes.", "Specific driver is different from the specific driver associated with the Logical Name.", "There is no session opened to the class driver.", "Max Error", "MAX - Error with config objects", "MAX - Error loading configuration", "MAX - Group not supported"]
        n119 = Format Into String(format string="Software Exception: Unhandled State \"%s\"." ("message"), w261) -> (resulting string=w256:string)  [unwired: 2 in, 1 out]
        n120 = call <userlib>:"Build Error Cluster__ogtk.vi"("String to Prepend to source (\"\")"=w256, "code"=w257) -> ("error out"=w255:errorcluster)
        n121 = call <vilib>:"Add State(s) to Queue__jki_lib_state_machine.vi"("State(s) in (\"\")"=w259) -> ("States Out"=w260:string)  [unwired: 14 in]
      }
      frame "Error Handler" {
        n122 = call-poly "Filter Error Codes__jki_lib_error_handling -- VI Tester.vi"("error in"=w268, "error codes to filter"=i32[] [1448, 74]) -> ("error out"=w267:errorcluster, "error filtered?"=w266:bool, "filtered error details"=w264:T15)  [unwired: 7 in]
        n123 = case shown="False" w266 {
          tunnel: w267 -> [w272 _]
          tunnel: w264 -> [_ w275]
          tunnel: w263 -> [_ w273]
          frame False {
            # "Very simple Error Handler"
            n124 = call <vilib>:"General Error Handler.vi"("error in (no error)"=w272) -> ()  [unwired: 10 in, 5 out]
          }
          frame True {
            n125 = Unbundle By Name(w275) -> ("code"=w274:i32)
            n126 = case shown="Default" w274 {
              selector: w274 -> [_ _ w284]
              tunnel: ["One or more tests or test harnesses has an invalid connector pane.  Missing Test reference." w278 w283] -> w276
              tunnel: w273 -> [_ w279 _]
              frame 74 {
              }
              frame 1448 {
                n127 = Unbundle By Name(w279) -> ("Test Project"=w280:path)
                n128 = Format Into String(format string="Error: Could not load classes from '%s'.\nMake sure 1+ classes inherit from testCase or testSuite." ("message"), w280) -> (resulting string=w278:string)  [unwired: 2 in, 1 out]
              }
              frame Default {
                n129 = Format Into String(format string="Filtered error '%d' has undefined message!", w284) -> (resulting string=w283:string)  [unwired: 2 in, 1 out]
              }
            }
            n130 = One Button Dialog(message=w276) -> ()  [unwired: 1 in, 1 out]
          }
        }
        n131 = call <vilib>:"Add State(s) to Queue__jki_lib_state_machine.vi"("State(s) in (\"\")"=w270) -> ("States Out"=w269:string)  [unwired: 14 in]
      }
      frame "Exit" {
        # "Generate Exit Event to stop bottom loop"
        n132 = Unbundle By Name(w290) -> ("Current VI's Refnum"=w289:refnum<vi>, "ExitEventReference"=w287:refnum<user-event>)
        n133 = Close Reference(reference=w289) -> (error out=w288:errorcluster)  [unwired: 1 in]
        n134 = Generate User Event(user event=w287, event data cluster=TRUE ("event data")) -> (error out=w286:errorcluster)  [unwired: 2 in, 1 out]
        n135 = call <vilib>:"Clear Errors.vi"("error in (no error)"=w288) -> ()  [unwired: 5 in, 2 out]
        n136 = call <vilib>:"Clear Errors.vi"("error in (no error)"=w286) -> ()  [unwired: 5 in, 2 out]
      }
      frame "Self Mass Compile" {
        # "LabVIEW IDE"
        # "packaged"
        n137 = call "Graphical Test Runner - Get Version.vi"() -> ("Dev. Environment?"=w304:bool)  [unwired: 4 in, 1 out]
        n138 = call "CheckForLabVIEW_IDE.vi"() -> ("LabVIEW IDE"=w301:bool)
        n139 = call "Read General Settings.vi"("error in"=w297) -> ("error out"=w296:errorcluster, "General"=w295:T14)  [unwired: 9 in]
        n140 = Not(x=w304) -> (.not. x?=w303:bool)
        n141 = Unbundle By Name(w295) -> ("SkipMassCompileCheck"=w294:bool)
        n142 = Compound Arithmetic op=AND(w303, w301, invert w294) -> (w302:bool)
        n143 = Unbundle By Name(w299) -> ("ProductName"=w298:string)
        n144 = case "Built?  Mass Compile" shown="True" w302 {
          tunnel: w296 -> [w306 w313]
          tunnel: [w306 w314] -> w300
          tunnel: w298 -> [_ w307]
          frame False {
          }
          frame True {
            # "Force the VI Tester project provider VI tree to load, so it gets\nnoticed by the Mass Compile Tool, then unload it afterwards."
            n145 = call <userlib>:"Application Directory__ogtk.vi"("Relative path (.)"=path "resource/JKI/VI Tester") -> ("Application Directory (+ Relative)"=w321:path)
            n146 = call <userlib>:"Application Directory__ogtk.vi"("Relative path (.)"=path "vi.lib/addons/_JKI Toolkits/VI Tester") -> ("Application Directory (+ Relative)"=w320:path)
            n147 = call <userlib>:"Application Directory__ogtk.vi"("Relative path (.)"=path "resource/Framework/Providers/vitester") -> ("Application Directory (+ Relative)"=w318:path)
            n148 = Build Path(base path=w318, name or relative path="VITester - VI Tree.vi") -> (appended path=w316:path)
            n149 = Build Array(w321, w320, w318) -> (w310:path[])
            n150 = Open VI Reference(vi path=w316, error in (no error)=w313) -> (vi reference=w315:refnum<vi>, error out=w309:errorcluster)  [unwired: 4 in]
            n151 = call "Mass Compile LabVIEW Tool__jki_lib_application_control -- VI Tester.vi"("error in (no error)"=w309, "Product Folders"=w310, "Product Name"=w307) -> ("error out"=w308:errorcluster)  [unwired: 8 in]
            n152 = call "Clear All Errors__jki_lib_error_handling -- VI Tester.vi"("error in"=w308) -> ("no error out"=w311:errorcluster)  [unwired: 4 in]
            n153 = Close Reference(reference=w315, error in (no error)=w311) -> (error out=w312:errorcluster)
            n154 = Merge Errors(w308, w312) -> (w314:errorcluster)
          }
        }
      }
      frame "---------- App Data ----------" {
        n155 = call <vilib>:"Add State(s) to Queue__jki_lib_state_machine.vi"("State(s) in (\"\")"=w325) -> ("States Out"=w324:string)  [unwired: 14 in]
      }
      frame "App Data: Cleanup" {
        n156 = Unbundle By Name(w331) -> ("TextStream"=w330:refnum<queue>)
        n157 = Release Queue(queue=w330, error in (no error)=w329) -> (error out=w328:errorcluster)  [unwired: 1 in, 2 out]
        n158 = call <vilib>:"Add State(s) to Queue__jki_lib_state_machine.vi"("State(s) in (\"\")"=w333) -> ("States Out"=w332:string)  [unwired: 14 in]
      }
      frame "App Data: Initialize" {
        # "if TestObject is wired, use it to load project"
        # "ignore error if project not used to launch UI"
        # "This should eventually use the same app context (reference) as the project (or app menu) that was used to launch the GUI Test Runner."
        n159 = property class="App"() -> (error out=w347:errorcluster, "Project.ActiveProject"=w349:refnum<vi>)  [unwired: 2 in, 1 out]
        n160 = Equal?(x="API_TestObject", y=refnum<class> refnum ("TestObject In")) -> (x = y?=w341:bool)
        n161 = call <vilib>:"Get LV Class Path.vi"("object"="API_TestObject") -> ("error out"=w340:errorcluster, "class path"=w339:path)  [unwired: 9 in]
        n162 = property class="Project"(reference=w349, error in=w347) -> (reference out=w348:refnum<vi>, error out=w346:errorcluster, "Path"=w338:path)
        n163 = call <vilib>:"Clear Errors.vi"("error in (no error)"=w340) -> ()  [unwired: 5 in, 2 out]
        n164 = control-ref of="This Application"() -> (w350:refnum<vi>)
        n165 = Close Reference(reference=w348, error in (no error)=w346) -> (error out=w345:errorcluster)
        n166 = Select(t=w338, s=w341, f=w339) -> (s? t:f=w336:path)
        n167 = call <vilib>:"Clear Errors.vi"("error in (no error)"=w345) -> ()  [unwired: 5 in, 2 out]
        n168 = control-ref of="This VI"() -> (w352:refnum<vi>)
        n169 = Current VI's Menubar() -> (w351:refnum<k9>)
        n170 = Bundle By Name(cluster=w343, "TestApplicationContext"=w350, "Current VI's Refnum"=w352, "menubar"=w351, "TextStream"=w344, "Test Project"=w336, "ProductName"="VI Tester") -> (w355:T6)
        n171 = call <vilib>:"Add State(s) to Queue__jki_lib_state_machine.vi"("State(s) in (\"\")"=w354) -> ("States Out"=w353:string)  [unwired: 14 in]
      }
      frame "---------- UI ----------" {
        n172 = call <vilib>:"Add State(s) to Queue__jki_lib_state_machine.vi"("State(s) in (\"\")"=w357) -> ("States Out"=w356:string)  [unwired: 14 in]
      }
      frame "UI: Set Busy" {
        w363 = TRUE  # animate?
        n173 = control-ref of="This VI"() -> (w362:refnum<vi>)
        n174 = control-ref of="Animated Throber"() -> (w365:refnum<vi>)
        n175 = control-ref of="Static Throber"() -> (w364:refnum<vi>)
        n176 = call <vilib>:"Set Busy.vi"("VI reference (current VI)"=w362) -> ("error out"=w360:errorcluster)  [unwired: 9 in, 1 out]
        n177 = call "Throber Control__jki_lib_user_interface -- VI Tester.vi"("animate?"=w363, "static throber reference"=w364, "animate throber reference"=w365) -> ()  [unwired: 9 in]
        n178 = call <vilib>:"Clear Errors.vi"("error in (no error)"=w360) -> ()  [unwired: 5 in, 2 out]
        n179 = call <vilib>:"Add State(s) to Queue__jki_lib_state_machine.vi"("State(s) in (\"\")"=w367) -> ("States Out"=w366:string)  [unwired: 14 in]
      }
      frame "UI: Set Free" {
        w372 = FALSE  # animate?
        n180 = control-ref of="Animated Throber"() -> (w374:refnum<vi>)
        n181 = control-ref of="Static Throber"() -> (w373:refnum<vi>)
        n182 = call "Throber Control__jki_lib_user_interface -- VI Tester.vi"("animate?"=w372, "static throber reference"=w373, "animate throber reference"=w374) -> ()  [unwired: 9 in]
        n183 = control-ref of="This VI"() -> (w371:refnum<vi>)
        n184 = call <vilib>:"Unset Busy.vi"("VI reference (current VI)"=w371) -> ("error out"=w370:errorcluster)  [unwired: 10 in]
        n185 = call <vilib>:"Clear Errors.vi"("error in (no error)"=w370) -> ()  [unwired: 5 in, 2 out]
        n186 = call <vilib>:"Add State(s) to Queue__jki_lib_state_machine.vi"("State(s) in (\"\")"=w376) -> ("States Out"=w375:string)  [unwired: 14 in]
      }
      frame "UI: Reset Tree Status" {
        n187 = Unbundle By Name(w385) -> ("TestTag"=w382:string)
        n188 = control-ref of="Test Hierarchy Tree"() -> (w384:refnum<vi>)
        n189 = call "Get All.vi"("Tree Reference In"=w384, "Starting Tag"=w382, "error in (no error)"=w383) -> ("Tree Reference Out"=w380:refnum<vi>, "Output Tree Items"=w381:string[], "error out"=w379:errorcluster)  [unwired: 13 in, 1 out]
        n190 = for {
          tunnel: w381 -> [w391] mode=indexing
          tunnel: w380 -> [w394]
          shift-right: [w392] -> w378
          shift-left: w379 -> [w393]
          n191 = Match Pattern(string=w391, regular expression=".lvclass") -> (offset past match=w389:i32)  [unwired: 1 in, 3 out]
          n192 = Less Or Equal To 0?(x=w389) -> (x <= 0?=w388:bool)
          n193 = case "Init Test Icon" shown="True" w388 {
            tunnel: w394 -> [_ w399]
            tunnel: w393 -> [w395 w398]
            tunnel: [w395 w397] -> w392
            tunnel: w391 -> [_ w396]
            frame False {
              # "leave class icon alone"
            }
            frame True {
              w400 = 39  # custom VI index
              n194 = property class="Tree"(reference=w399, error in=w398, "Active Item Tag"=w396, "Glyph"=w400) -> (error out=w397:errorcluster)  [unwired: 1 out]
            }
          }
        }
        n195 = call <vilib>:"Add State(s) to Queue__jki_lib_state_machine.vi"("State(s) in (\"\")"=w387) -> ("States Out"=w386:string)  [unwired: 14 in]
      }
      frame "UI: Init Tree Symbols" {
        n196 = invoke on="Test Hierarchy Tree" class="Tree (strict)" method="Custom Item Symbols.Revert Symbols"() -> (error out=w403:errorcluster)  [unwired: 3 in, 2 out]
        n197 = call "Get Tree Symbols.vi"() -> ("Tree Symbols"=w401:T16[])  [unwired: 11 in]
        n198 = invoke on="Test Hierarchy Tree" class="Tree (strict)" method="Custom Item Symbols.Set Symbol Array"(error in=w403, "glyphs"=w401) -> ()  [unwired: 2 in, 4 out]
        n199 = call <vilib>:"Add State(s) to Queue__jki_lib_state_machine.vi"("State(s) in (\"\")"=w405) -> ("States Out"=w404:string)  [unwired: 14 in]
      }
      frame "UI: Interlock" {
        # "abort is only enabled when testSuite.run invoked"
        n200 = Unbundle By Name(w438) -> ("TestRunning"=w412:bool, "InitializingTree"=w407:bool)
        n201 = property on="Test Hierarchy Tree" class="Tree (strict)"() -> ("DispItems"=w434:string[])  [unwired: 2 in, 2 out]
        n202 = local read "Detailed Status"() -> (w414:string)
        n203 = property on="Test Hierarchy Tree" class="Tree (strict)"() -> ("DispItems"=w418:string[], "Value"=w417:string)  [unwired: 2 in, 2 out]
        n204 = Not(x=w407) -> (.not. x?=w422:bool)
        n205 = Not(x=w412) -> (.not. x?=w424:bool)
        n206 = property on="Abort" class="Bool"("Disabled"=enum16{"enabled", "disabled", "grayed out"}."grayed out") -> ()  [unwired: 2 in, 2 out]
        n207 = Empty String/Path?(string/path=w414) -> (empty?=w413:bool)
        n208 = Array Size(array=w418) -> (size(s)=w419:i32)
        n209 = Empty String/Path?(string/path=w417) -> (empty?=w416:bool)
        n210 = Greater Than 0?(x=w419) -> (x > 0?=w415:bool)
        n211 = Array Size(array=w434) -> (size(s)=w433:i32)
        n212 = Compound Arithmetic op=AND(invert w407, invert w412, invert w413) -> (w411:bool)
        n213 = Compound Arithmetic op=AND(w415, invert w416) -> (w437:bool)
        n214 = Greater Than 0?(x=w433) -> (x > 0?=w425:bool)
        n215 = Select(t=T8."Enabled" ("Disabled"), s=w411, f=T8."Disabled and Grayed Out" ("Disabled")) -> (s? t:f=w408:T8)
        n216 = Compound Arithmetic op=AND(w425, w424, w422) -> (w421:bool)
        n217 = Compound Arithmetic op=AND(w422, w424, w437) -> (w436:bool)
        n218 = Compound Arithmetic op=AND(w424, w422) -> (w423:bool)
        n219 = property on="Save Report" class="Bool"("DisabledEnum"=w408) -> ()  [unwired: 2 in, 2 out]
        n220 = Select(t=T8."Enabled" ("Disabled"), s=w436, f=T8."Disabled and Grayed Out" ("Disabled")) -> (s? t:f=w439:T8)
        n221 = Select(t=T8."Enabled" ("Disabled"), s=w423, f=T8."Disabled and Grayed Out" ("Disabled")) -> (s? t:f=w428:T8)
        n222 = Select(t=T8."Enabled" ("Disabled"), s=w421, f=T8."Disabled and Grayed Out" ("Disabled")) -> (s? t:f=w420:T8)
        n223 = property on="Run Single Test" class="Bool"("DisabledEnum"=w439) -> ()  [unwired: 2 in, 2 out]
        n224 = property on="Reload" class="Bool"("DisabledEnum"=w428) -> ()  [unwired: 2 in, 2 out]
        n225 = property on="Run All" class="Bool"("DisabledEnum"=w420) -> ()  [unwired: 2 in, 2 out]
        n226 = property on="Collapse Tree" class="Bool"("DisabledEnum"=w420) -> ()  [unwired: 2 in, 2 out]
        n227 = property on="Expand Tree" class="Bool"("DisabledEnum"=w420) -> ()  [unwired: 2 in, 2 out]
        n228 = call <vilib>:"Add State(s) to Queue__jki_lib_state_machine.vi"("State(s) in (\"\")"=w441) -> ("States Out"=w440:string)  [unwired: 14 in]
      }
      frame "UI: Front Panel State" {
        n229 = Unbundle By Name(w445) -> ("Current VI's Refnum"=w443:refnum<vi>)
        n230 = case shown="\"Open\", Default" w444 {
          tunnel: w443 -> [w449 w452]
          frame "Open", Default {
            n231 = invoke class="VI" method="FP.Open"(reference=w449, "Activate"=TRUE, "State"=T9."Standard") -> ()  [unwired: 2 in, 5 out]
          }
          frame "Close" {
            n232 = invoke class="VI" method="FP.Close"(reference=w452) -> ()  [unwired: 2 in, 3 out]
          }
        }
        n233 = call <vilib>:"Add State(s) to Queue__jki_lib_state_machine.vi"("State(s) in (\"\")"=w447) -> ("States Out"=w446:string)  [unwired: 14 in]
      }
      frame "UI: Initialize" {
        w457 = "0" ("txtFailures:")
        w456 = ""
        w463 = TRUE  # Delete All?
        # "flush report queue whenever UI is initialized"
        n234 = Flush Queue(queue=w453) -> ()  [unwired: 1 in, 3 out]
        n235 = property on="Test Hierarchy Tree" class="Tree (strict)"("ActiveColNum"=u32 1 ("Number of Columns"), "Width"=3000 ("Active Cell:Cell Size:Width")) -> ()  [unwired: 2 in, 2 out]
        n236 = local write "txtPassed:"(w457) -> ()
        n237 = local write "txtSkipped"(w457) -> ()
        n238 = local write "txtRuns:"(w457) -> ()
        n239 = local write "txtFailed:"(w457) -> ()
        n240 = control-ref of="Slide"() -> (w459:refnum<vi>)
        n241 = invoke on="Test Hierarchy Tree" class="Tree (strict)" method="Edit Tree Items.Delete"("Delete Children"=w463) -> ()  [unwired: 4 in, 5 out]
        n242 = local write "Test Hierarchy Tree"(w456) -> ()
        n243 = local write "Detailed Status"(w456) -> ()
        n244 = call "UpdateFailbar.vi"("Function"=FailbarStatus--Enum."Initialize", "Slide Refnum"=w459) -> ()  [unwired: 10 in]
        n245 = call <vilib>:"Add State(s) to Queue__jki_lib_state_machine.vi"("State(s) in (\"\")"=w465) -> ("States Out"=w466:string)  [unwired: 14 in]
        "Animated Throber" <- T2 0 ("Animated Throber")
        "Static Throber" <- T1 0 ("Static Throber")
        "Slide" <- u8 100 ("FailureBar")
      }
      frame "UI: Uninitialize" {
        w471 = "0" ("txtFailures:")
        w475 = TRUE  # Delete All?
        n246 = local write "Animated Throber"(T2 0 ("Animated Throber")) -> ()
        n247 = local write "Static Throber"(T1 0 ("Static Throber")) -> ()
        n248 = local write "Slide"(u8 0 ("FailureBar")) -> ()
        n249 = local write "txtPassed:"(w471) -> ()
        n250 = local write "txtSkipped"(w471) -> ()
        n251 = local write "txtRuns:"(w471) -> ()
        n252 = local write "txtFailed:"(w471) -> ()
        n253 = control-ref of="Slide"() -> (w473:refnum<vi>)
        n254 = invoke on="Test Hierarchy Tree" class="Tree (strict)" method="Edit Tree Items.Delete"("Delete Children"=w475) -> ()  [unwired: 4 in, 5 out]
        n255 = local write "Detailed Status"("") -> ()
        n256 = call "UpdateFailbar.vi"("Function"=FailbarStatus--Enum."Initialize", "Slide Refnum"=w473) -> ()  [unwired: 10 in]
        n257 = call <vilib>:"Add State(s) to Queue__jki_lib_state_machine.vi"("State(s) in (\"\")"=w477) -> ("States Out"=w478:string)  [unwired: 14 in]
      }
      frame "UI: Open File Dialog" {
        n258 = Unbundle By Name(w482) -> ("StartTestTime"=w483:timestamp)
        n259 = Unbundle By Name(w482) -> ("Test Project"=w488:path)
        n260 = Not Equal?(x=timestamp(0 s since 1904-01-01) ("y"), y=w483) -> (x != y?=w485:bool)
        n261 = case "Test results exist" shown="True" w485 {
          tunnel: [TRUE ("T button?") w504] -> w486
          frame False {
          }
          frame True {
            n262 = Two Button Dialog(message="Changing the path will clear the current results.") -> (T button?=w504:bool)  [unwired: 2 in]
          }
        }
        n263 = case "show file dialog" shown="True" w486 {
          tunnel: [TRUE ("T button?") w498] -> w491
          tunnel: "LabVIEW Project or Class" ("message") -> [_ w501]
          tunnel: w488 -> [w495 w500]
          tunnel: [w495 w499] -> w489
          tunnel: "Select LabVIEW Project or Class" ("message") -> [_ w497]
          frame False {
          }
          frame True {
            n264 = call "File Dialog__jki_lib_file -- VI Tester.vi"("start path"=w500, "prompt"=w497, "pattern label"=w501, "pattern"="*.lvproj;*.lvclass" ("message")) -> ("path"=w499:path, "cancelled"=w498:bool)  [unwired: 8 in, 2 out]
          }
        }
        n265 = case "cancelled" shown="False" w491 {
          tunnel: w482 -> [w510 w511]
          tunnel: [w509 w511] -> w481
          tunnel: w489 -> [w508 _]
          tunnel: ["UI: Set Busy\nUI: Update Title\nMacro: Load Tree\nUI: Set Free" ("message") _] -> w480
          frame False {
            # "initialize UI since no tests of the new\npath have been run"
            n266 = Bundle By Name(cluster=w510, "Test Project"=w508, "StartTestTime"=timestamp(0 s since 1904-01-01)) -> (w509:T6)
          }
          frame True {
            # "reset path to previous path"
          }
        }
        n267 = call <vilib>:"Add State(s) to Queue__jki_lib_state_machine.vi"("State(s) in Front (\"\")"=w480, "State(s) in (\"\")"=w492) -> ("States Out"=w493:string)  [unwired: 13 in]
      }
      frame "UI: Update Title" {
        w519 = "%s - %s"  # expected title
        n268 = Unbundle By Name(w522) -> ("Current VI's Refnum"=w521:refnum<vi>, "Test Project"=w520:path, "ProductName"=w512:string)
        n269 = Strip Path(path=w520) -> (name=w513:string)  [unwired: 1 out]
        n270 = Format Into String(format string=w519, w512, w513) -> (resulting string=w517:string)  [unwired: 2 in, 1 out]
        n271 = Empty String/Path?(string/path=w513) -> (empty?=w518:bool)
        n272 = Select(t=w512, s=w518, f=w517) -> (s? t:f=w516:string)
        n273 = property class="VI"(reference=w521, error in=w515, "Front Panel.Title"=w516) -> (error out=w514:errorcluster)  [unwired: 1 out]
        n274 = call <vilib>:"Add State(s) to Queue__jki_lib_state_machine.vi"("State(s) in (\"\")"=w523) -> ("States Out"=w524:string)  [unwired: 14 in]
      }
      frame "---------- Panel ----------" {
        n275 = call <vilib>:"Add State(s) to Queue__jki_lib_state_machine.vi"("State(s) in (\"\")"=w526) -> ("States Out"=w525:string)  [unwired: 14 in]
      }
      frame "Panel: Open" {
        # "Open VI Front Panel"
        n276 = Unbundle By Name(w533) -> ("TestApplicationContext"=w529:refnum<vi>, "Open Path"=w534:path)
        n277 = Unbundle By Name(w533) -> ("Test Project"=w532:path)
        n278 = call-poly <userlib>:"Strip Path Extension__ogtk.vi"("path"=w534) -> ("extension"=w535:string)  [unwired: 1 out]
        n279 = case shown="\"vi\"" w535 {
          selector: w535 -> [w541 _ _]
          tunnel: w534 -> [_ w557 w568]
          tunnel: w532 -> [_ _ w571]
          tunnel: w531 -> [w538 w556 w561]
          tunnel: [w539 w545 w570] -> w530
          tunnel: w529 -> [_ w544 w560]
          frame Default {
            w543 = 1 items=["No error", "Argument error", "Memory is full", "Out of zone", "End of file", "File already open", "Generic file I/O error", "File not found", "File permission error", "Disk is full", "Duplicate path", "Too many files open", "System feature not enabled", "Resource file not found", "Cannot add resource", "Resource not found", "Image not found", "Image memory error", "Pen does not exist", "Config type invalid", "Config token not found", "Config parse error", "Config memory error", "Bad external code format", "Bad external code offset", "External code not present", "Null window", "Destroy window error", "Null menu", "Print aborted", "Bad print record", "Print driver error", "Windows error during printing", "Memory error during printing", "Print dialog error", "Generic print error", "Invalid device refnum", "Device not found", "Device parameter error", "Device unit error", "Cannot open device", "Device call aborted", "Generic error", "Cancelled by user", "Object ID too low", "Object ID too high", "Object not in heap", "Unknown heap", "Unknown object (invalid DefProc)", "Unknown object (DefProc not in table)", "Message out of range", "Invalid (null) method", "Unknown message", "Manager call not supported", "Bad address", "Network operation in progress", "Network operation timed out", "Connection is busy", "Network attribute not supported", "Network error", "Address in use", "System out of memory", "Connection aborted", "Connection refused", "Not connected", "Already connected", "Connection closed", "Initialization error (interapplication manager)", "Bad occurrence", "Wait on unbound occurrence handler", "Occurrence queue overflow", "Datalog type conflict", "Unused", "Unrecognized type (interapplication manager)", "Memory corrupt", "Failed to make temporary DLL", "Old CIN version", "Drag socket not found", "Failed to load drop-object", "Failed to register OLE object", "Failed to release OLE object", "Format specifier type mismatch", "Unknown format specifier", "Too few format specifiers", "Too many format specifiers", "Scan failed", "Newer CIN version", "Error converting to variant", "Runtime menu error", "Password tampered", "Variant attribute not found", "Incompatible variant data type", "Event data is not available", "Event Store is not present", "Occurrence is not found", "Event Queue is not created", "Event info is not available", "Refnum passed is NULL", "Error retrieving Class GUID", "Error retrieving CoClass GUID", "Error retrieving TypeLib GUID.", "Bad built application magic bytes.", "Specific driver is different from the specific driver associated with the Logical Name.", "There is no session opened to the class driver.", "Max Error", "MAX - Error with config objects", "MAX - Error loading configuration", "MAX - Group not supported"]
            n280 = Format Into String(format string="Invalid file type '.%s'", w541) -> (resulting string=w540:string)  [unwired: 2 in, 1 out]
            n281 = call <vilib>:"Error Cluster From Error Code.vi"("error in (no error)"=w538, "error message (\"\")"=w540, "error code (0)"=w543) -> ("error out"=w539:errorcluster)  [unwired: 6 in]
          }
          frame "lvclass" {
            n282 = invoke class="App" method="Library.Open"(reference=w544, error in=w556, "path"=w557) -> (reference out=w549:refnum<vi>, error out=w552:errorcluster, "Open Library"=w555:refnum<vi>)  [unwired: 1 in, 1 out]
            n283 = property class="Library"(reference=w555, error in=w552) -> (reference out=w550:refnum<vi>, error out=w553:errorcluster, "Project"=w554:refnum<vi>)
            n284 = invoke class="Project" method="Open Window"(reference=w554, error in=w553) -> (reference out=w551:refnum<vi>, error out=w546:errorcluster)  [unwired: 1 in, 1 out]
            n285 = Close Reference(reference=w551, error in (no error)=w546) -> (error out=w548:errorcluster)
            n286 = Close Reference(reference=w550, error in (no error)=w548) -> (error out=w547:errorcluster)
            n287 = Close Reference(reference=w549, error in (no error)=w547) -> (error out=w545:errorcluster)
          }
          frame "vi" {
            # "Try to open VI as if its in memory, if that errors then open it from disk"
            n288 = Strip Path(path=w571) -> (name=w577:string)  [unwired: 1 out]
            n289 = Strip Path(path=w568) -> (name=w576:string)  [unwired: 1 out]
            n290 = Format Into String(format string="%s:%s", w577, w576) -> (resulting string=w562:string)  [unwired: 2 in, 1 out]
            n291 = Open VI Reference(application reference (local)=w560, vi path=w562, error in (no error)=w561) -> (vi reference=w558:refnum<vi>, error out=w559:errorcluster)  [unwired: 3 in]
            n292 = case "Open from disk" shown="Error" w559 {
              selector: w559 -> [w579 w584]
              tunnel: [w583 w584] -> w573
              tunnel: [w582 w585] -> w572
              tunnel: w568 -> [w581 _]
              tunnel: w560 -> [w580 _]
              tunnel: w558 -> [_ w585]
              frame Error {
                n293 = call <vilib>:"Clear Errors.vi"("error in (no error)"=w579) -> ("error out"=w578:errorcluster)  [unwired: 5 in, 1 out]
                n294 = Open VI Reference(application reference (local)=w580, vi path=w581, error in (no error)=w578) -> (vi reference=w582:refnum<vi>, error out=w583:errorcluster)  [unwired: 3 in]
              }
              frame No Error {
              }
            }
            n295 = invoke class="VI" method="FP.Open"(reference=w572, error in=w573, "Activate"=TRUE ("Activate?"), "State"=T9."Standard") -> (reference out=w564:refnum<vi>, error out=w566:errorcluster)  [unwired: 1 in, 3 out]
            n296 = property class="VI"(reference=w564, error in=w566, "Front Panel.IsFrontmost"=TRUE ("Front Panel Window:Is Frontmost")) -> (reference out=w563:refnum<vi>, error out=w565:errorcluster)
            n297 = Close Reference(reference=w563, error in (no error)=w565) -> (error out=w570:errorcluster)
          }
        }
        n298 = call <vilib>:"Add State(s) to Queue__jki_lib_state_machine.vi"("State(s) in (\"\")"=w537) -> ("States Out"=w536:string)  [unwired: 14 in]
      }
      frame "---------- Test ----------" {
        n299 = call <vilib>:"Add State(s) to Queue__jki_lib_state_machine.vi"("State(s) in (\"\")"=w587) -> ("States Out"=w586:string)  [unwired: 14 in]
      }
      frame "Test: Run Result Handler" {
        w602 = T17 {"txtRuns"=refnum, "txtSkipped"=refnum, "txtFailures"=refnum, "txtPassed"=refnum, "txtSimple Status"=refnum, "Test Hierarchy Tree"=refnum}  # TestRunner_UI_Refs
        n300 = control-ref of="Test Hierarchy Tree"() -> (w593:refnum<vi>)
        n301 = control-ref of="txtRuns:"() -> (w601:refnum<vi>)
        n302 = control-ref of="txtSkipped"() -> (w597:refnum<vi>)
        n303 = control-ref of="txtFailed:"() -> (w596:refnum<vi>)
        n304 = control-ref of="txtPassed:"() -> (w595:refnum<vi>)
        n305 = control-ref of="Simple Status"() -> (w594:refnum<vi>)
        n306 = Unbundle By Name(w600) -> ("ResultChangedRef"=w606:refnum<user-event>, "SuiteChangedRef"=w605:refnum<user-event>, "ExitEventReference"=w604:refnum<user-event>, "AbortEventRef"=w607:refnum<user-event>, "TestStartedEventRef"=w590:refnum<user-event>)
        n307 = Bundle By Name(cluster=w602, "txtRuns"=w601, "txtSkipped"=w597, "txtFailures"=w596, "txtPassed"=w595, "txtSimple Status"=w594, "Test Hierarchy Tree"=w593) -> (w603:T17)
        n308 = Bundle By Name(cluster=T11 {"ResultStatusChanged"=refnum, "SuiteStatusChanged"=refnum, "Exit"=refnum, "Abort"=refnum, "TestStartedEventRef"=refnum} ("TestStatusEvents"), "ResultStatusChanged"=w606, "SuiteStatusChanged"=w605, "Exit"=w604, "Abort"=w607, "TestStartedEventRef"=w590) -> (w591:T11)
        n309 = call "Dynamic Results Status Update Process.vi"("error in (no error)"=w599, "TestStatusEvents"=w591, "TestRunner_UI_Refs"=w603) -> ("error out"=w598:errorcluster)  [unwired: 8 in]
        n310 = call <vilib>:"Add State(s) to Queue__jki_lib_state_machine.vi"("State(s) in (\"\")"=w609) -> ("States Out"=w608:string)  [unwired: 14 in]
      }
      frame "Test: Load Methods" {
        n311 = call <vilib>:"Add State(s) to Queue__jki_lib_state_machine.vi"("State(s) in (\"\")"=w613) -> ("States Out"=w612:string)  [unwired: 14 in]
      }
      frame "Test: Load Hierarchy" {
        w625 = ""
        n312 = control-ref of="Test Hierarchy Tree"() -> (w624:refnum<vi>)
        n313 = call "Dynamic Load and Execute Tests Process.vi"("API_TextTestRunner"=w615, "error in"=w616, "App Data"=w614, "Operation"=enum16{"Load", "Run Test", "Run All Tests"}."Load", "Test Hierarchy Tree"=w624) -> ("error out"=w621:errorcluster, "Tree Methods"=w623:i32)  [unwired: 5 in]
        n314 = Select(t="", s=w621, f="Project: Store Path") -> (s? t:f=w618:string)
        n315 = Bundle By Name(cluster=w614, "TotalTests"=w623, "Last Failure"=w625, "Last Tree Value"=w625, "InitializingTree"=FALSE) -> (w626:T6)
        n316 = call <vilib>:"Add State(s) to Queue__jki_lib_state_machine.vi"("State(s) in Front (\"\")"=w618, "State(s) in (\"\")"=w628) -> ("States Out"=w627:string)  [unwired: 13 in]
      }
      frame "Test: Start" {
        # "Valid refnum"
        n317 = Flush Queue(queue=w635) -> ()  [unwired: 1 in, 3 out]
        n318 = Not A Number/Path/Refnum?(number/path/refnum=w631) -> (NaN/Path/Refnum?=w634:bool)
        n319 = Not(x=w634) -> (.not. x?=w633:bool)
        n320 = case "Fire TestStatusChanged" shown="True" w633 {
          tunnel: "Running" ("spreadsheet string") -> [_ w650]
          tunnel: w631 -> [_ w649]
          tunnel: w630 -> [w646 w648]
          tunnel: [w646 w647] -> w629
          frame False {
          }
          frame True {
            n321 = Generate User Event(user event=w649, event data cluster=w650, error in=w648) -> (error out=w647:errorcluster)  [unwired: 1 in, 1 out]
          }
        }
        n322 = Get Date/Time In Seconds() -> (seconds since 1Jan1904=w640:timestamp)
        n323 = Bundle By Name(cluster=w645, "StartTestTime"=w640, "TestRunning"=TRUE) -> (w642:T6)
        n324 = control-ref of="Animated Throber"() -> (w639:refnum<vi>)
        n325 = control-ref of="Static Throber"() -> (w638:refnum<vi>)
        n326 = call "Throber Control__jki_lib_user_interface -- VI Tester.vi"("animate?"=TRUE, "static throber reference"=w638, "animate throber reference"=w639) -> ()  [unwired: 9 in]
        n327 = call "UpdateFailbar.vi"("Function"=FailbarStatus--Enum."Start") -> ()  [unwired: 11 in]
        n328 = call <vilib>:"Add State(s) to Queue__jki_lib_state_machine.vi"("State(s) in (\"\")"=w644) -> ("States Out"=w643:string)  [unwired: 14 in]
      }
      frame "Test: Initialize UI" {
        w651 = "0" ("Errors:")
        # "clear errors"
        n329 = local write "Simple Status"(w657) -> ()
        n330 = Unbundle By Name(w655) -> ("TotalTests"=w654:i32)
        n331 = local write "Detailed Status"("") -> ()
        n332 = Format Into String(format string="0/%d", w654) -> (resulting string=→"txtRuns:":string)  [unwired: 2 in, 1 out]
        n333 = call <vilib>:"Add State(s) to Queue__jki_lib_state_machine.vi"("State(s) in (\"\")"=w659) -> ("States Out"=w658:string)  [unwired: 14 in]
        "txtPassed:" <- w651
        "txtFailed:" <- w651
        "txtSkipped" <- w651
      }
      frame "Test: Run Test Tag" {
        # "Run selected tests based on tree or failures tab"
        n334 = property on="Abort" class="Bool"(error in=w666, "DisabledEnum"=T8."Enabled" ("Disabled")) -> (error out=w661:errorcluster)  [unwired: 1 in, 1 out]
        n335 = control-ref of="Test Hierarchy Tree"() -> (w663:refnum<vi>)
        n336 = call "Dynamic Load and Execute Tests Process.vi"("API_TextTestRunner"=w665, "error in"=w661, "App Data"=w668, "Operation"=enum16{"Load", "Run Test", "Run All Tests"}."Run Test", "Test Hierarchy Tree"=w663) -> ("error out"=w667:errorcluster)  [unwired: 5 in, 1 out]
        n337 = call <vilib>:"Add State(s) to Queue__jki_lib_state_machine.vi"("State(s) in (\"\")"=w670) -> ("States Out"=w669:string)  [unwired: 14 in]
      }
      frame "Test: Run All Tests" {
        n338 = control-ref of="Test Hierarchy Tree"() -> (w674:refnum<vi>)
        n339 = property on="Abort" class="Bool"(error in=w675, "Disabled"=enum16{"enabled", "disabled", "grayed out"}."enabled") -> (error out=w676:errorcluster)  [unwired: 1 in, 1 out]
        n340 = call "Dynamic Load and Execute Tests Process.vi"("API_TextTestRunner"=w672, "error in"=w676, "App Data"=w673, "Operation"=enum16{"Load", "Run Test", "Run All Tests"}."Run All Tests", "Test Hierarchy Tree"=w674) -> ("error out"=w678:errorcluster)  [unwired: 5 in, 1 out]
        n341 = call <vilib>:"Add State(s) to Queue__jki_lib_state_machine.vi"("State(s) in (\"\")"=w680) -> ("States Out"=w679:string)  [unwired: 14 in]
      }
      frame "Test: Update Results" {
        w696 = TRUE  # return elements?
        # "Valid refnum"
        # "Valid refnum"
        # "update Simple Status with timing details"
        n342 = Not A Number/Path/Refnum?(number/path/refnum=w684) -> (NaN/Path/Refnum?=w686:bool)
        n343 = Not(x=w686) -> (.not. x?=w685:bool)
        n344 = case "Fire TestStatusChanged" shown="True" w685 {
          tunnel: "Idle" ("spreadsheet string") -> [_ w709]
          tunnel: w684 -> [_ w708]
          tunnel: w682 -> [w705 w707]
          tunnel: [w705 w706] -> w681
          frame False {
          }
          frame True {
            n345 = Generate User Event(user event=w708, event data cluster=w709, error in=w707) -> (error out=w706:errorcluster)  [unwired: 1 in, 1 out]
          }
        }
        n346 = Unbundle By Name(w702) -> ("StartTestTime"=w699:timestamp)
        n347 = Get Date/Time In Seconds() -> (seconds since 1Jan1904=w700:timestamp)
        n348 = Get Queue Status(queue=w692, return elements? (F)=w696) -> (elements=w695:string[])  [unwired: 1 in, 7 out]
        n349 = Subtract(x=w700, y=w699) -> (x-y=w698:dbl)
        n350 = Array To Spreadsheet String(delimiter (Tab)="\r\n", array=w695, 3:"%s" ("format string")) -> (spreadsheet string=w691:string)
        n351 = Format Into String(format string="Finished: %.2f seconds", w698) -> (resulting string=→"Simple Status":string)  [unwired: 2 in, 1 out]
        n352 = Not A Number/Path/Refnum?(number/path/refnum="API_CompleteTestReport") -> (NaN/Path/Refnum?=w689:bool)
        n353 = Not(x=w689) -> (.not. x?=w687:bool)
        n354 = case "Fire TestReportChanged" shown="True" w687 {
          tunnel: w691 -> [_ w714]
          tunnel: "API_CompleteTestReport" -> [_ w713]
          tunnel: w681 -> [w710 w712]
          tunnel: [w710 w711] -> w688
          frame False {
          }
          frame True {
            n355 = Generate User Event(user event=w713, event data cluster=w714, error in=w712) -> (error out=w711:errorcluster)  [unwired: 1 in, 1 out]
          }
        }
        n356 = call <vilib>:"Add State(s) to Queue__jki_lib_state_machine.vi"("State(s) in (\"\")"=w704) -> ("States Out"=w703:string)  [unwired: 14 in]
      }
      frame "Test: Stop" {
        # "clean up temp test objects"
        n357 = control-ref of="Animated Throber"() -> (w719:refnum<vi>)
        n358 = control-ref of="Static Throber"() -> (w718:refnum<vi>)
        n359 = call "Throber Control__jki_lib_user_interface -- VI Tester.vi"("static throber reference"=w718, "animate throber reference"=w719) -> ()  [unwired: 10 in]
        n360 = call "UpdateFailbar.vi"("Progress"=u32 100, "Function"=FailbarStatus--Enum."Update Progress") -> ()  [unwired: 10 in]
        n361 = Bundle By Name(cluster=w715, "TestRunning"=FALSE) -> (w721:T6)
        n362 = call <vilib>:"Add State(s) to Queue__jki_lib_state_machine.vi"("State(s) in (\"\")"=w723) -> ("States Out"=w722:string)  [unwired: 14 in]
      }
      frame "---------- Project ----------" {
        n363 = call <vilib>:"Add State(s) to Queue__jki_lib_state_machine.vi"("State(s) in (\"\")"=w726) -> ("States Out"=w725:string)  [unwired: 14 in]
      }
      frame "Project: Store Path" {
        n364 = Unbundle By Name(w732) -> ("Test Project"=w731:path)
        n365 = call "Prepend Test Project Path If New.vi"("error in"=w730, "Test Project"=w731) -> ("error out"=w729:errorcluster)  [unwired: 9 in]
        n366 = call <vilib>:"Add State(s) to Queue__jki_lib_state_machine.vi"("State(s) in (\"\")"=w734) -> ("States Out"=w733:string)  [unwired: 14 in]
      }
      frame "Project: Open" {
        n367 = String To Path(string=w743) -> (path=w736:path)
        n368 = call-poly <userlib>:"Strip Path Extension__ogtk.vi"("path"=w736) -> ("extension"=w741:string)  [unwired: 1 out]
        n369 = case "check file type" shown="\"\"" w741 {
          tunnel: w740 -> [w746 w749 w752 w755]
          tunnel: [w746 w748 w751 w754] -> w738
          tunnel: w736 -> [_ w747 w750 w753]
          frame Default {
          }
          frame "lvclass" {
            n370 = Bundle By Name(cluster=w749, "Test Project"=w747, "Test Class"=w747) -> (w748:T6)
          }
          frame "lvproj" {
            n371 = Bundle By Name(cluster=w752, "Test Project"=w750) -> (w751:T6)
          }
          frame "" {
            n372 = Bundle By Name(cluster=w755, "Test Project"=w753) -> (w754:T6)
          }
        }
        n373 = Bundle By Name(cluster=w738, "TestTag"="") -> (w737:T6)
        n374 = call <vilib>:"Add State(s) to Queue__jki_lib_state_machine.vi"("State(s) in Front (\"\")"="Macro: Load Tree" ("State(s) in Front (\"\")"), "State(s) in (\"\")"=w745) -> ("States Out"=w744:string)  [unwired: 13 in]
      }
      frame "Project: Get Tests" {
        # "do not support tests outside of testCase objects"
        # "get tests that aren't members of test Classes"
      }
      frame "Project: Get Classes" {
        # "sort alphabetically"
        # "Discover Test objects (TestCase and TestSuite class ancestors)"
        n375 = Unbundle By Name(w766) -> ("Test Project"=w765:path)
        n376 = call-poly <userlib>:"Strip Path Extension__ogtk.vi"("path"=w765) -> ("extension"=w764:string)  [unwired: 1 out]
        n377 = case "Load Project from lvproj file" shown="\"lvproj\"" w764 {
          tunnel: w769 -> [w780 w790]
          tunnel: [w776 w789] -> w767
          tunnel: w765 -> [w781 w788]
          tunnel: [w772 w787] -> w760
          frame Default {
            w774 = string[] ["TestCase.lvclass", "TestSuite.lvclass"]  # Framework classes
            # "load from folder -- find all *.lvclass that are not part of the framework"
            n378 = call <userlib>:"List Directory Recursive__ogtk.vi"("error in (no error)"=w780, "pattern"="*.lvclass", "Path"=w781) -> ("error out"=w776:errorcluster, "file paths"=w777:path[])  [unwired: 5 in, 2 out]
            n379 = call-poly <userlib>:"Strip Path__ogtk.vi"("path"=w777) -> ("name"=w779:string[])  [unwired: 1 out]
            n380 = call-poly <userlib>:"Filter 1D Array__ogtk.vi"("items to filter"=w774, "array"=w779) -> ("filtered item indices"=w778:i32[])  [unwired: 4 in, 1 out]
            n381 = call-poly <userlib>:"Delete Elements from Array__ogtk.vi"("indices"=w778, "array"=w777) -> ("array w/ subset deleted"=w773:path[])  [unwired: 8 in, 1 out]
            n382 = for {
              tunnel: w773 -> [w786] mode=indexing
              tunnel: w776 -> [w785]
              tunnel: [w784] -> w775 mode=indexing
              n383 = call "Check if Path Is Test Class.vi"("error in"=w785, "Test Class Path"=w786) -> ("error out"=w783:errorcluster, "IsTestObject"=w784:bool)  [unwired: 7 in, 1 out]
              n384 = call <vilib>:"Clear Errors.vi"("error in (no error)"=w783) -> ()  [unwired: 5 in, 2 out]
            }
            n385 = call-poly <userlib>:"Conditional Auto-Indexing Tunnel__ogtk.vi"("Array in"=w773, "Elements to keep"=w775) -> ("Filtered Array out"=w772:path[])  [unwired: 5 in]
          }
          frame "lvproj" {
            n386 = call "Find Project Test Objects.vi"("error in"=w790, "Project"=w788) -> ("error out"=w789:errorcluster, "TestPaths"=w787:path[])  [unwired: 8 in]
          }
        }
        n387 = call-poly <userlib>:"Strip Path__ogtk.vi"("path"=w760) -> ("name"=w763:string[])  [unwired: 1 out]
        n388 = call-poly <userlib>:"Sort Array__ogtk.vi"("Order"=enum16{"ascending", "descending"}."ascending", "Array in"=w763) -> ("Sorted Pointers"=w761:i32[])  [unwired: 8 in, 1 out]
        n389 = call-poly <userlib>:"Index Array Elements__ogtk.vi"("indices"=w761, "array"=w760) -> ("elements"=w759:path[])  [unwired: 9 in]
        n390 = Bundle By Name(cluster=w766, "TestProjectClasses"=w759) -> (w768:T6)
        n391 = call <vilib>:"Add State(s) to Queue__jki_lib_state_machine.vi"("State(s) in (\"\")"=w771) -> ("States Out"=w770:string)  [unwired: 14 in]
      }
      frame "Project: Get Class" {
        # "Get Tests from Test Object"
        # "TestType"
        # "IsTest"
        # "For now, discard non-Test Case classes... in future, will inspect any class for tests"
        n392 = Unbundle By Name(w801) -> ("Test Project"=w794:path)
        n393 = call "Check if Path Is Test Class.vi"("error in"=w793, "Test Class Path"=w794) -> ("error out"=w796:errorcluster, "TestType"=w795:string, "IsTestObject"=w797:bool)  [unwired: 7 in]
        n394 = call "Clear All Errors__jki_lib_error_handling -- VI Tester.vi"("error in"=w796) -> ()  [unwired: 4 in, 1 out]
        n395 = case shown="\"TestSuite\"" w795 {
          tunnel: w794 -> [_ w807]
          tunnel: w793 -> [w805 w809]
          tunnel: [w805 w808] -> w792
          tunnel: [_ w806] -> w791
          frame Default {
          }
          frame "TestSuite" {
            # "find all project classes\nwithin TestSuite"
            n396 = call "Dynamic Get TestSuite Test Paths.vi"("error in"=w809, "Test Project"=w807) -> ("error out"=w808:errorcluster, "Test Paths"=w806:path[])  [unwired: 8 in]
          }
        }
        n397 = Select(t=w794, s=w797, f=path "") -> (s? t:f=w799:path)
        n398 = Build Array (concatenate)(w799, w791) -> (w798:path[])
        n399 = Bundle By Name(cluster=w801, "TestProjectClasses"=w798) -> (w802:T6)
        n400 = call <vilib>:"Add State(s) to Queue__jki_lib_state_machine.vi"("State(s) in (\"\")"=w804) -> ("States Out"=w803:string)  [unwired: 14 in]
      }
      frame "---------- Macro ----------" {
        n401 = call <vilib>:"Add State(s) to Queue__jki_lib_state_machine.vi"("State(s) in (\"\")"=w811) -> ("States Out"=w810:string)  [unwired: 14 in]
      }
      frame "Macro: Load Tree" {
        # "cancelled"
        n402 = Unbundle By Name(w826) -> ("Test Project"=w815:path)
        n403 = call <userlib>:"Strip Path Extension - Path__ogtk.vi"("path"=w815) -> ("extension"=w825:string)  [unwired: 1 out]
        n404 = case shown="\"\", \"lvproj\"" w825 {
          selector: w825 -> [w830 _ _]
          tunnel: [_ "Project: Get Class\nProject: Get Tests" ("State(s) in Front") "Project: Get Classes\nProject: Get Tests" ("State(s) in Front")] -> w822
          tunnel: [w829 _ _] -> w816
          frame Default {
            n405 = Format Into String(format string="Invalid Project Type '%s'", w830) -> (resulting string=w831:string)  [unwired: 2 in, 1 out]
            n406 = One Button Dialog(message=w831) -> (true=w829:bool)  [unwired: 1 in]
          }
          frame "lvclass" {
          }
          frame "", "lvproj" {
          }
        }
        n407 = Not(x=w816) -> (.not. x?=w817:bool)
        n408 = Bundle By Name(cluster=w826, "InitializingTree"=w817) -> (w818:T6)
        n409 = call <vilib>:"Add State(s) to Queue__jki_lib_state_machine.vi"("State(s) in Front (\"\")"="UI: Interlock\nUI: Initialize\nUI: Update Title\nTest: Initialize UI >> Scanning for tests ..." ("State(s) in Front"), "State(s) in (\"\")"=w822, "State(s) at Back (\"\")"="Test: Load Hierarchy\nTest: Update Results\nTest: Initialize UI >> Ready\nUI: Interlock" ("State(s) in Front")) -> ("States Out"=w821:string)  [unwired: 12 in]
        n410 = Select(t="", s=w816, f=w821) -> (s? t:f=w820:string)
        n411 = call <vilib>:"Add State(s) to Queue__jki_lib_state_machine.vi"("State(s) in Front (\"\")"=w820, "State(s) in (\"\")"=w828) -> ("States Out"=w827:string)  [unwired: 13 in]
      }
      frame "Macro: Initialize" {
        n412 = call <vilib>:"Add State(s) to Queue__jki_lib_state_machine.vi"("State(s) in Front (\"\")"="Test: Initialize UI >> Initializing ...\nApp Data: Initialize\nUI: Update Title\nUI: Initialize\nUI: Init Tree Symbols\nUI: Front Panel State >> Open\nSelf Mass Compile\nUI: Set Busy\nMacro: Load Tree\nUI: Set Free" ("State(s) in Front"), "State(s) in (\"\")"=w837) -> ("States Out"=w836:string)  [unwired: 13 in]
      }
      frame "Macro: Start Test" {
        n413 = call <vilib>:"Add State(s) to Queue__jki_lib_state_machine.vi"("State(s) in Front (\"\")"="UI: Reset Tree Status\nTest: Start\nUI: Interlock\nTest: Initialize UI >> Running ..." ("State(s) in Front"), "State(s) in (\"\")"=w842) -> ("States Out"=w841:string)  [unwired: 13 in]
      }
      frame "Macro: Run All Tests" {
        # "Run all tests loaded on tree"
        n414 = call <vilib>:"Add State(s) to Queue__jki_lib_state_machine.vi"("State(s) in Front (\"\")"="Macro: Start Test\nTest: Run Result Handler\nTest: Run All Tests\nMacro: Stop Test", "State(s) in (\"\")"=w847) -> ("States Out"=w846:string)  [unwired: 13 in]
      }
      frame "Macro: Run Test Tag" {
        n415 = Unbundle By Name(w855) -> ("TestTag"=w854:string)
        n416 = call "Insert Test Loader Cases.vi"("TestTag"=w854) -> ("Cases to Insert"=w851:string)
        n417 = call <vilib>:"Add State(s) to Queue__jki_lib_state_machine.vi"("State(s) in Front (\"\")"="Macro: Start Test", "State(s) in (\"\")"=w851, "State(s) at Back (\"\")"="Test: Run Result Handler\nTest: Run Test Tag\nMacro: Stop Test") -> ("States Out"=w850:string)  [unwired: 12 in]
        n418 = call <vilib>:"Add State(s) to Queue__jki_lib_state_machine.vi"("State(s) in Front (\"\")"=w850, "State(s) in (\"\")"=w857) -> ("States Out"=w856:string)  [unwired: 13 in]
      }
      frame "Macro: Stop Test" {
        n419 = call <vilib>:"Add State(s) to Queue__jki_lib_state_machine.vi"("State(s) in Front (\"\")"="Test: Stop\nTest: Update Results\nUI: Interlock", "State(s) in (\"\")"=w861) -> ("States Out"=w860:string)  [unwired: 13 in]
      }
      frame "Macro: Exit" {
        # "Built?"
        n420 = call "Graphical Test Runner - Get Version.vi"() -> ("Dev. Environment?"=w870:bool)  [unwired: 4 in, 1 out]
        n421 = Not(x=w870) -> (.not. x?=w869:bool)
        n422 = Select(t="UI: Front Panel State >> Close" ("State(s) in Front"), s=w869, f="") -> (s? t:f=w867:string)
        n423 = call <vilib>:"Add State(s) to Queue__jki_lib_state_machine.vi"("State(s) in Front (\"\")"=w867, "State(s) at Back (\"\")"="UI: Uninitialize\nApp Data: Cleanup\nExit" ("State(s) in Front")) -> ("States Out"=w865:string)  [unwired: 13 in]
        n424 = call <vilib>:"Add State(s) to Queue__jki_lib_state_machine.vi"("State(s) in Front (\"\")"=w865, "State(s) in (\"\")"=w872) -> ("States Out"=w871:string)  [unwired: 13 in]
      }
      frame "---------- Help ----------" {
        n425 = call <vilib>:"Add State(s) to Queue__jki_lib_state_machine.vi"("State(s) in (\"\")"=w876) -> ("States Out"=w875:string)  [unwired: 14 in]
      }
      frame "Help: Example Project" {
        w880 = path "examples/JKI/VI Tester/VI Tester Example.lvproj"  # installed example project path
        n426 = Unbundle By Name(w884) -> ("StartTestTime"=w885:timestamp)
        n427 = Not Equal?(x=timestamp(0 s since 1904-01-01) ("y"), y=w885) -> (x != y?=w887:bool)
        n428 = case "Test results exist" shown="True" w887 {
          tunnel: [TRUE ("T button?") w892] -> w881
          frame False {
          }
          frame True {
            n429 = Two Button Dialog(message="Changing the path will clear the current results.") -> (T button?=w892:bool)  [unwired: 2 in]
          }
        }
        n430 = call <userlib>:"Application Directory__ogtk.vi"("Relative path (.)"=w880) -> ("Application Directory (+ Relative)"=w879:path)
        n431 = case "cancelled" shown="True" w881 {
          tunnel: w884 -> [w894 w899]
          tunnel: [w894 w898] -> w883
          tunnel: [_ "UI: Update Title\nMacro: Load Tree" ("message")] -> w882
          tunnel: w879 -> [_ w895]
          frame False {
            # "reset path to previous path"
          }
          frame True {
            # "initialize UI since no tests of the new\npath have been run"
            n432 = Bundle By Name(cluster=w899, "Test Project"=w895, "StartTestTime"=timestamp(0 s since 1904-01-01)) -> (w898:T6)
          }
        }
        n433 = call <vilib>:"Add State(s) to Queue__jki_lib_state_machine.vi"("State(s) in Front (\"\")"=w882, "State(s) in (\"\")"=w889) -> ("States Out"=w888:string)  [unwired: 13 in]
      }
      frame "---------- Results ----------" {
        n434 = call <vilib>:"Add State(s) to Queue__jki_lib_state_machine.vi"("State(s) in (\"\")"=w901) -> ("States Out"=w900:string)  [unwired: 14 in]
      }
      frame "Results: Print" {
        w904 = 43 items=["No error", "Argument error", "Memory is full", "Out of zone", "End of file", "File already open", "Generic file I/O error", "File not found", "File permission error", "Disk is full", "Duplicate path", "Too many files open", "System feature not enabled", "Resource file not found", "Cannot add resource", "Resource not found", "Image not found", "Image memory error", "Pen does not exist", "Config type invalid", "Config token not found", "Config parse error", "Config memory error", "Bad external code format", "Bad external code offset", "External code not present", "Null window", "Destroy window error", "Null menu", "Print aborted", "Bad print record", "Print driver error", "Windows error during printing", "Memory error during printing", "Print dialog error", "Generic print error", "Invalid device refnum", "Device not found", "Device parameter error", "Device unit error", "Cannot open device", "Device call aborted", "Generic error", "Cancelled by user", "Object ID too low", "Object ID too high", "Object not in heap", "Unknown heap", "Unknown object (invalid DefProc)", "Unknown object (DefProc not in table)", "Message out of range", "Invalid (null) method", "Unknown message", "Manager call not supported", "Bad address", "Network operation in progress", "Network operation timed out", "Connection is busy", "Network attribute not supported", "Network error", "Address in use", "System out of memory", "Connection aborted", "Connection refused", "Not connected", "Already connected", "Connection closed", "Initialization error (interapplication manager)", "Bad occurrence", "Wait on unbound occurrence handler", "Occurrence queue overflow", "Datalog type conflict", "Unused", "Unrecognized type (interapplication manager)", "Memory corrupt", "Failed to make temporary DLL", "Old CIN version", "Drag socket not found", "Failed to load drop-object", "Failed to register OLE object", "Failed to release OLE object", "Format specifier type mismatch", "Unknown format specifier", "Too few format specifiers", "Too many format specifiers", "Scan failed", "Newer CIN version", "Error converting to variant", "Runtime menu error", "Password tampered", "Variant attribute not found", "Incompatible variant data type", "Event data is not available", "Event Store is not present", "Occurrence is not found", "Event Queue is not created", "Event info is not available", "Refnum passed is NULL", "Error retrieving Class GUID", "Error retrieving CoClass GUID", "Error retrieving TypeLib GUID.", "Bad built application magic bytes.", "Specific driver is different from the specific driver associated with the Logical Name.", "There is no session opened to the class driver.", "Max Error", "MAX - Error with config objects", "MAX - Error loading configuration", "MAX - Group not supported"]
        n435 = local read "Detailed Status"() -> (w908:string)
        n436 = call <vilib>:"Easy Text Report.vi"("text to be printed"=w908, "error in (no error)"=w907) -> ("error out"=w906:errorcluster)  [unwired: 13 in]
        n437 = call-poly "Filter Error Codes__jki_lib_error_handling -- VI Tester.vi"("error in"=w906, "error code to filter"=w904) -> ("error out"=w905:errorcluster)  [unwired: 7 in, 2 out]
        n438 = call <vilib>:"Add State(s) to Queue__jki_lib_state_machine.vi"("State(s) in (\"\")"=w910) -> ("States Out"=w909:string)  [unwired: 14 in]
      }
      frame "Results: Save" {
        # "cancelled"
        n439 = Unbundle By Name(w915) -> ("ProductName"=w914:string)
        n440 = Format Into String(format string="%s.txt", w914) -> (resulting string=w916:string)  [unwired: 2 in, 1 out]
        n441 = Concatenate Strings("%Y_%m_%d_%H_%M_%S " ("time format string (%c)"), w916) -> (w912:string)
        n442 = Format Date/Time String(time format string (%c)=w912) -> (date/time string=w923:string)  [unwired: 2 in]
        n443 = call "File Dialog__jki_lib_file -- VI Tester.vi"("prompt"="Save Results As ...", "selection mode (existing file)"=T12."new or existing file", "pattern label"="Text file; All files", "default name"=w923, "pattern"="*.txt; *.*" ("pattern label")) -> ("path"=w920:path, "cancelled"=w922:bool)  [unwired: 7 in, 2 out]
        n444 = Not(x=w922) -> (.not. x?=w921:bool)
        n445 = case shown="True" w921 {
          tunnel: w920 -> [_ w936]
          tunnel: w919 -> [w930 w935]
          tunnel: [w930 w932] -> w918
          frame False {
          }
          frame True {
            w931 = TRUE  # convert eol? (no:F)
            w934 = 43 items=["No error", "Argument error", "Memory is full", "Out of zone", "End of file", "File already open", "Generic file I/O error", "File not found", "File permission error", "Disk is full", "Duplicate path", "Too many files open", "System feature not enabled", "Resource file not found", "Cannot add resource", "Resource not found", "Image not found", "Image memory error", "Pen does not exist", "Config type invalid", "Config token not found", "Config parse error", "Config memory error", "Bad external code format", "Bad external code offset", "External code not present", "Null window", "Destroy window error", "Null menu", "Print aborted", "Bad print record", "Print driver error", "Windows error during printing", "Memory error during printing", "Print dialog error", "Generic print error", "Invalid device refnum", "Device not found", "Device parameter error", "Device unit error", "Cannot open device", "Device call aborted", "Generic error", "Cancelled by user", "Object ID too low", "Object ID too high", "Object not in heap", "Unknown heap", "Unknown object (invalid DefProc)", "Unknown object (DefProc not in table)", "Message out of range", "Invalid (null) method", "Unknown message", "Manager call not supported", "Bad address", "Network operation in progress", "Network operation timed out", "Connection is busy", "Network attribute not supported", "Network error", "Address in use", "System out of memory", "Connection aborted", "Connection refused", "Not connected", "Already connected", "Connection closed", "Initialization error (interapplication manager)", "Bad occurrence", "Wait on unbound occurrence handler", "Occurrence queue overflow", "Datalog type conflict", "Unused", "Unrecognized type (interapplication manager)", "Memory corrupt", "Failed to make temporary DLL", "Old CIN version", "Drag socket not found", "Failed to load drop-object", "Failed to register OLE object", "Failed to release OLE object", "Format specifier type mismatch", "Unknown format specifier", "Too few format specifiers", "Too many format specifiers", "Scan failed", "Newer CIN version", "Error converting to variant", "Runtime menu error", "Password tampered", "Variant attribute not found", "Incompatible variant data type", "Event data is not available", "Event Store is not present", "Occurrence is not found", "Event Queue is not created", "Event info is not available", "Refnum passed is NULL", "Error retrieving Class GUID", "Error retrieving CoClass GUID", "Error retrieving TypeLib GUID.", "Bad built application magic bytes.", "Specific driver is different from the specific driver associated with the Logical Name.", "There is no session opened to the class driver.", "Max Error", "MAX - Error with config objects", "MAX - Error loading configuration", "MAX - Group not supported"]
            n446 = local read "Detailed Status"() -> (w937:string)
            n447 = call "Write Characters to File - With Error in and Error Out - __jki_lib_file -- VI Tester.vi"("file path (dialog if empty)"=w936, "character string"=w937, "error in (no error)"=w935, "convert eol? (no:F)"=w931) -> ("error out"=w933:errorcluster)  [unwired: 10 in, 1 out]
            n448 = call-poly "Filter Error Codes__jki_lib_error_handling -- VI Tester.vi"("error in"=w933, "error code to filter"=w934) -> ("error out"=w932:errorcluster)  [unwired: 7 in, 2 out]
          }
        }
        n449 = call <vilib>:"Add State(s) to Queue__jki_lib_state_machine.vi"("State(s) in (\"\")"=w929) -> ("States Out"=w928:string)  [unwired: 14 in]
      }
      frame "---------- For Expansion ----------" {
        n450 = call <vilib>:"Add State(s) to Queue__jki_lib_state_machine.vi"("State(s) in (\"\")"=w939) -> ("States Out"=w938:string)  [unwired: 14 in]
      }
    }
  }
  n451 = while "Status Event Loop (checks for all status related data)" {
    tunnel: w24 -> [w949]
    tunnel: w22 -> [w948]
    tunnel: [w947] -> w21
    shift-right: [w945] -> _
    shift-left: w18 -> [w946]
    tunnel: 100 -> [w944]
    tunnel: w13 -> [w943]
    tunnel: "API_TesterStatus" -> [w942]
    stop <- w950 stop-if-true
    n452 = event shown="[2] \"Abort\": Value Change" {
      selector: w948 -> [_ _ _]
      dyn-events: [_ _ _] -> w947
      timeout: w944 -> [_ _ _]
      tunnel: [_ TRUE _] -> w950
      tunnel: w949 -> [w957 _ _]
      tunnel: w946 -> [w956 w968 w978]
      tunnel: [w956 w968 w978] -> w945
      tunnel: w943 -> [_ _ w975]
      tunnel: w942 -> [_ _ w969]
      event Timeout {
        n453 = event-data() -> ()  [unwired: 1 in, 2 out]
        n454 = Get Queue Status(queue=w957) -> (queue out=w951:refnum<queue>, error out=w953:errorcluster, # elements in queue=w955:i32)  [unwired: 2 in, 5 out]
        n455 = call-poly <userlib>:"Data Changed__ogtk.vi"("I32"=w955) -> ("Changed"=w954:bool)
        n456 = case "Stream changed" shown="True" w954 {
          tunnel: w953 -> [w958 w964]
          tunnel: [w958 w961] -> w952
          tunnel: w951 -> [_ w960]
          frame False {
          }
          frame True {
            w962 = TRUE  # return elements?
            n457 = Get Queue Status(queue=w960, return elements? (F)=w962, error in (no error)=w964) -> (error out=w961:errorcluster, elements=w963:string[])  [unwired: 6 out]
            n458 = Array To Spreadsheet String(delimiter (Tab)="\r\n", array=w963, 3:"%s" ("format string")) -> (spreadsheet string=→"Detailed Status":string)
          }
        }
        n459 = call <vilib>:"Clear Errors.vi"("error in (no error)"=w952) -> ()  [unwired: 5 in, 2 out]
      }
      event User Event {
        # "Exit Loop"
        n460 = event-data() -> ()  [unwired: 1 in, 5 out]
      }
      event "Abort": Value Change {
        # "Valid refnum"
        n461 = event-data() -> ()  [unwired: 1 in, 6 out]
        n462 = Generate User Event(user event=w975, event data cluster=TRUE ("event data")) -> (error out=w976:errorcluster)  [unwired: 2 in, 1 out]
        n463 = call <vilib>:"Clear Errors.vi"("error in (no error)"=w976) -> ()  [unwired: 5 in, 2 out]
        n464 = Not A Number/Path/Refnum?(number/path/refnum=w969) -> (NaN/Path/Refnum?=w972:bool)
        n465 = Not(x=w972) -> (.not. x?=w971:bool)
        n466 = case "Fire TestStatusChanged" shown="True" w971 {
          tunnel: "Aborting" ("spreadsheet string") -> [_ w980]
          tunnel: w969 -> [_ w979]
          frame False {
          }
          frame True {
            n467 = Generate User Event(user event=w979, event data cluster=w980) -> ()  [unwired: 2 in, 2 out]
          }
        }
        n468 = local write "Simple Status"("Aborting ..." ("Simple Status")) -> ()
        n469 = property on="Abort" class="Bool"("Disabled"=enum16{"enabled", "disabled", "grayed out"}."grayed out") -> ()  [unwired: 2 in, 2 out]
      }
    }
  }
  n470 = Unregister For Events(event registration refnum=w21) -> (error out=w20:errorcluster)  [unwired: 1 in]
  n471 = Destroy User Event(user event=w6, error in=w20) -> (error out=w15:errorcluster)
  n472 = Destroy User Event(user event=w5, error in=w15) -> (error out=w14:errorcluster)
  n473 = Destroy User Event(user event=w13, error in=w14) -> (error out=w11:errorcluster)
  n474 = Destroy User Event(user event=w10, error in=w11) -> ()  [unwired: 1 out]
